vi "Off Mode Standby Mode Power Measure SM.vi"(0 "Aplus IP Address":string="192.168.1.101", 5 "Remote Port":i32=502, 11 "Error In":errorcluster) -> (2 "Complete?":bool, 4 "Off Mode Watts":dbl, 6 "2015 Output":bool, 8 "Standby Watts":dbl, 10 "Low Power Switch":bool=TRUE, 15 "Error Out":errorcluster)   [LabVIEW 2012]
uses:
  <vilib>/Analysis/NI_AALBase.lvlib
panel:
  in  "Main Tab":enum32{"Collecting", "Analyzed"}(tab)
  in  "stop":bool
  out "Power Chart":dbl(graph)
  out "Power (Watts)":dbl format="%#.2g"
  in  "Skip Standby":bool
  in  "2015 DOE":bool
  out "Off Mode Watts":T1(graph)
  out "5% of Max.":dbl
  out "Max Value.":dbl
  out "Standard Deviation.":dbl
  out "Standby Mode Watts":T1(graph)
  out "Standard Deviation":dbl
  out "Max Value":dbl
  out "5% of Max":dbl
  in  "Complete Test":bool
  in  "Restart":bool
  out "Stable?":bool
  out "Time Sum 4":dbl
  out "Time Sum 3":dbl
  out "Time Sum 2":dbl
  out "Time Sum 1":dbl
  in  "Tab Control":enum32{"Input Parameters", "Debug", "Raw Data"}(tab)
  in  "Processed Data":bool
  in  "Tab Control 2":T2(tab)
  in  "10 Min Power":dbl=600.0
  in  "35 Min":dbl=2100.0
  in  "5 Min Timer":dbl=300.0
  in  "2015?":bool
  out "Current State":string
  in  "High State Timer":dbl=10.0
  out "High Power":dbl
  in  "Low State Timer (5 min)":dbl=300.0
  out "Power Threshold":dbl
  in  "Testing":bool
  in  "Test Power":dbl
  in  "Debug?":bool=TRUE
  out "Debug State":string[](array[string])
  out "DOE Data":dbl[][](array[numeric])
  out "35 Min Data":dbl[][](array[numeric])
  out "Power Threshold Array":dbl[][](array[numeric])
  out "Timer":dbl format="%<%H:%M:%S>t"
  out "String":string
  # "Measure off mode and standby mode for DOE 2015. Reference ETP 112D026 - 2015 DOE Dryer Energy"
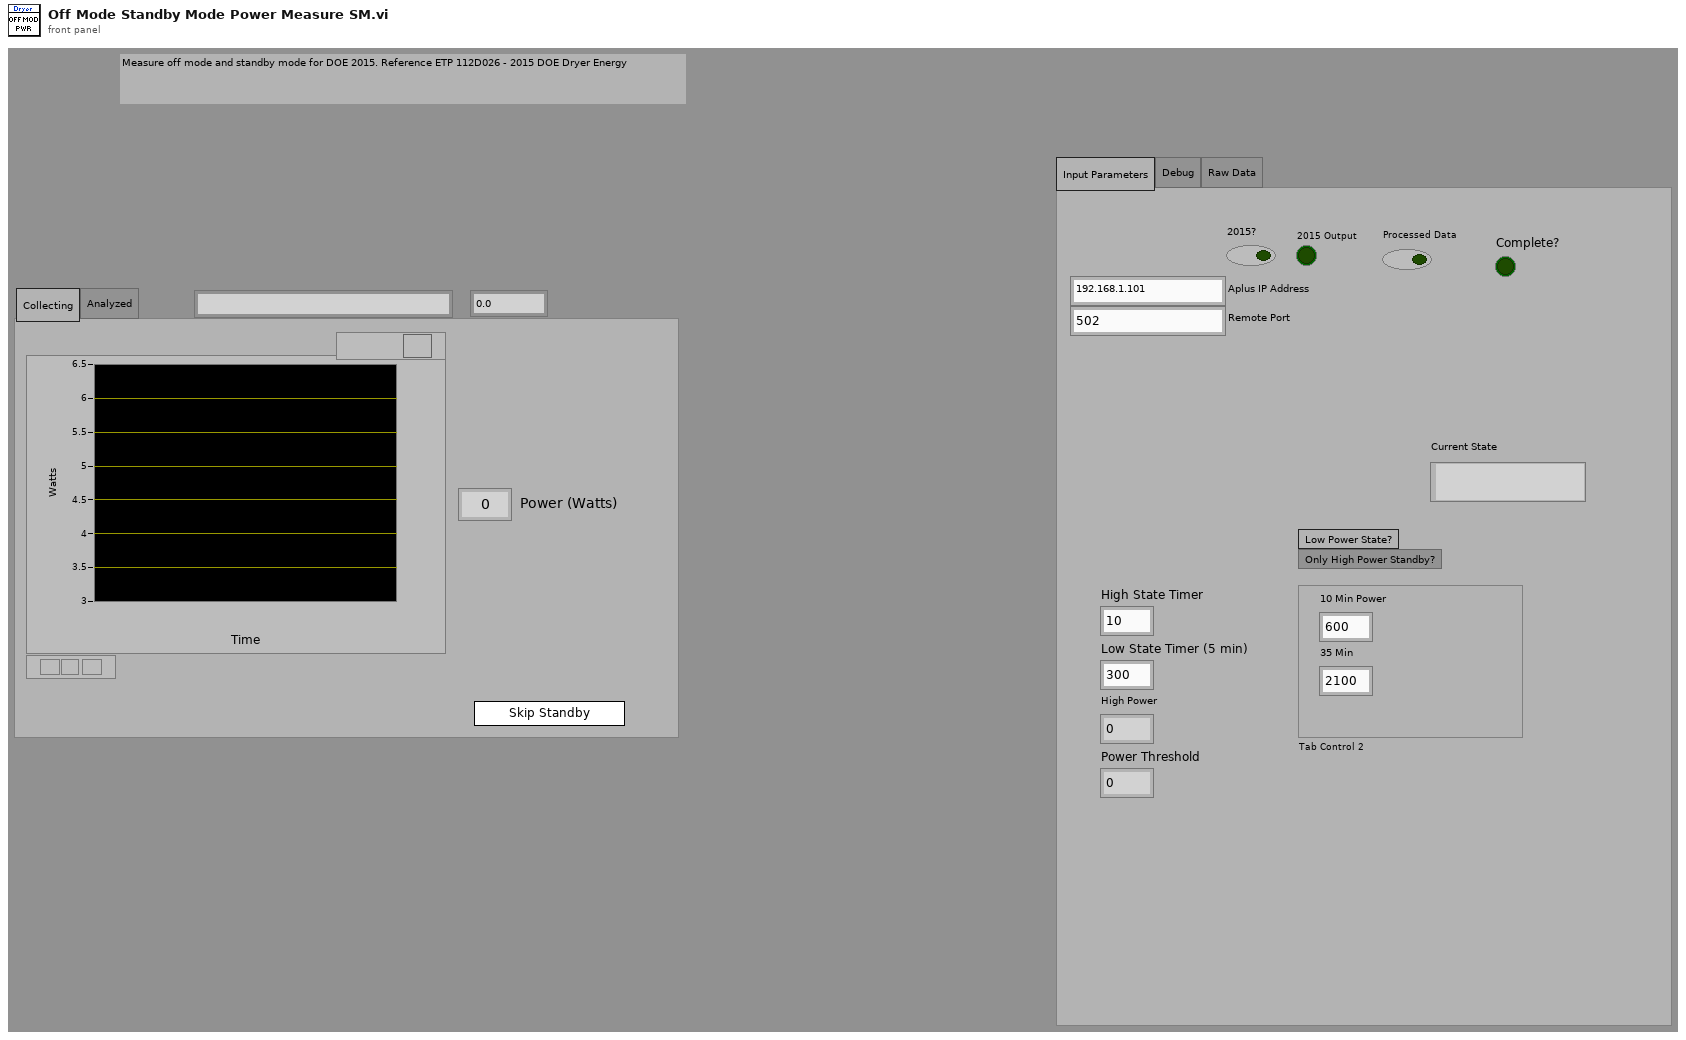
[diagram p1: front panel]
types:
  T1 = cluster{"X Values":dbl[], "Histogram: h(x)":i32[]}
  T2 = enum32{"Low Power State?", "Only High Power Standby?"}
  T3 = enum32{"invalid app kind", "Development System", "Run Time System", "Student Edition", "Embedded LabVIEW", "Evaluation", "Custom"}
  T4 = enum32{"Invalid", "Standard", "Closed", "Hidden", "Minimized", "Maximized"}
  T5 = cluster{"Core":cluster{"Current VI Reference":refnum<vi>, "Close Panel on Exit?":bool}, "Agilent Channel List":string, "T0":dbl, "Tstart":dbl, "Temps":dbl[], "2015?":bool, "Labels":string[], "35 Min Data Array":dbl[], "10 Min Data Array":dbl[], "Low Power State?":bool, "Output Data":cluster{"Standard Deviation":dbl, "Off Mode Watts":dbl, "Max Value":dbl, "5% of Max":dbl, "Standby Watts":dbl, "Standard Deviation.":dbl, "Max Value.":dbl, "5% of Max.":dbl}, "Power Threshold":dbl[], "Processed Data":bool, "Main Tab":enum32{"Collecting", "Analyzed"}, "Remote Port":i32, "Aplus IP Address":string}
  T6 = cluster{"Standard Deviation":dbl, "Off Mode Watts":dbl, "Max Value":dbl, "5% of Max":dbl, "Standby Watts":dbl, "Standard Deviation.":dbl, "Max Value.":dbl, "5% of Max.":dbl}
  T7 = cluster{"Current VI Reference":refnum<vi>, "Close Panel on Exit?":bool}
  T8 = cluster{"Voltage":sgl, "Current":sgl, "Frequency":sgl, "Power":sgl, "Power Factor":sgl, "WattHours":sgl}
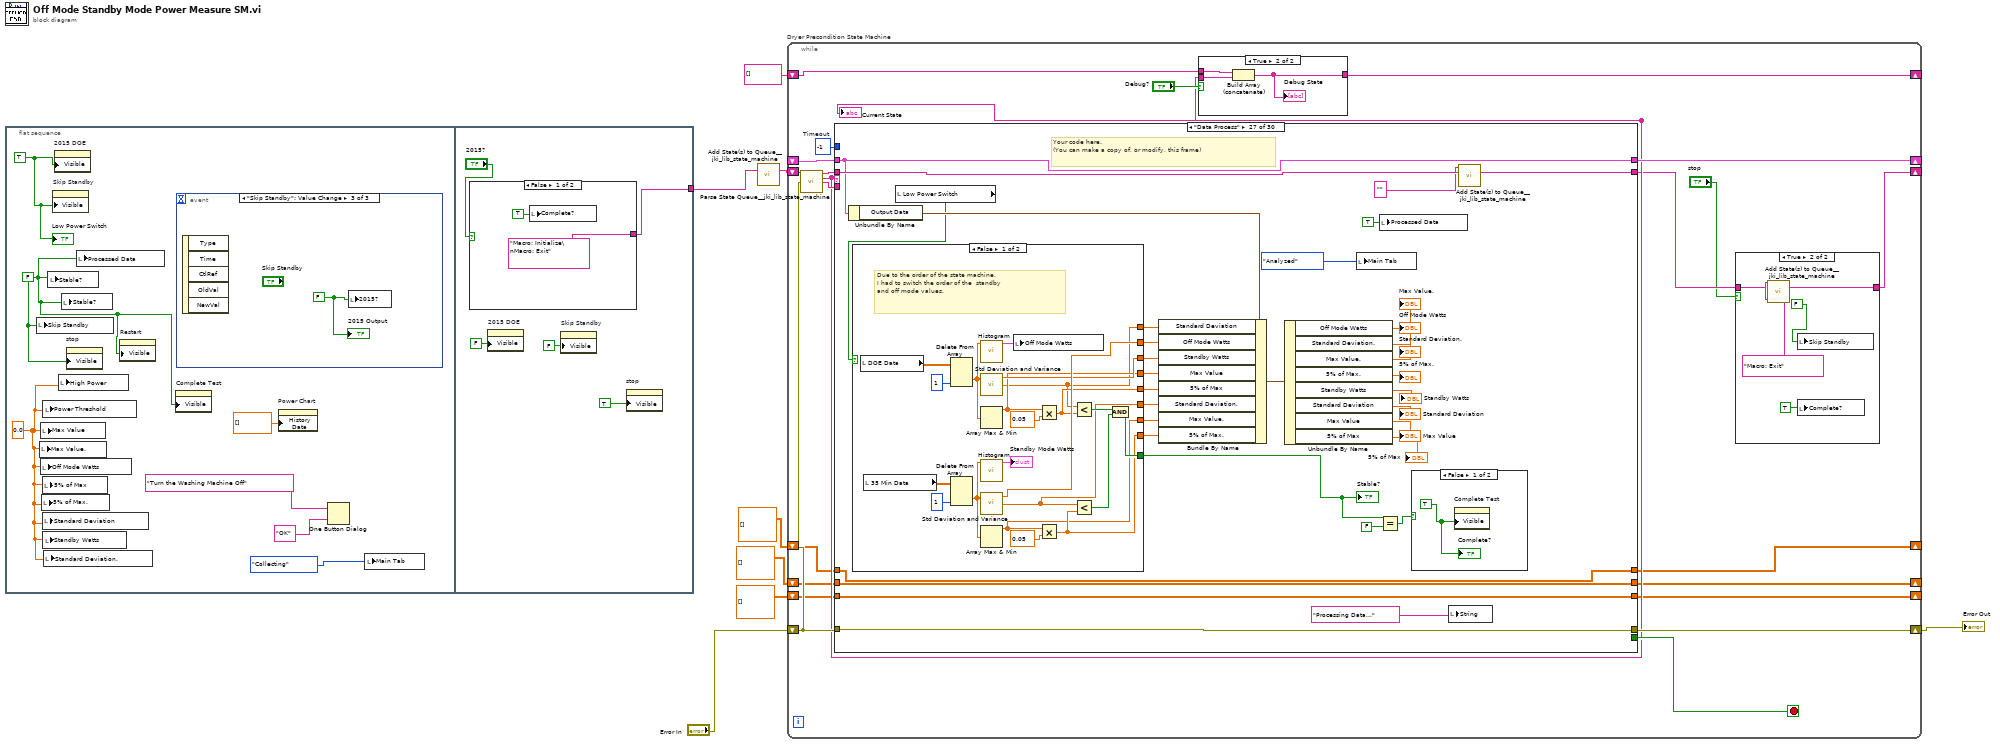
[diagram p0: block diagram]
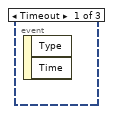
[diagram p2: hidden frame]
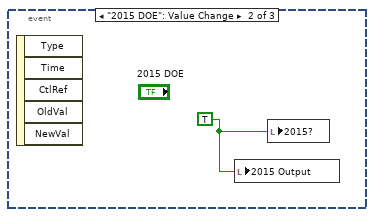
[diagram p3: hidden frame]
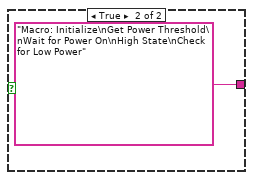
[diagram p4: hidden frame]
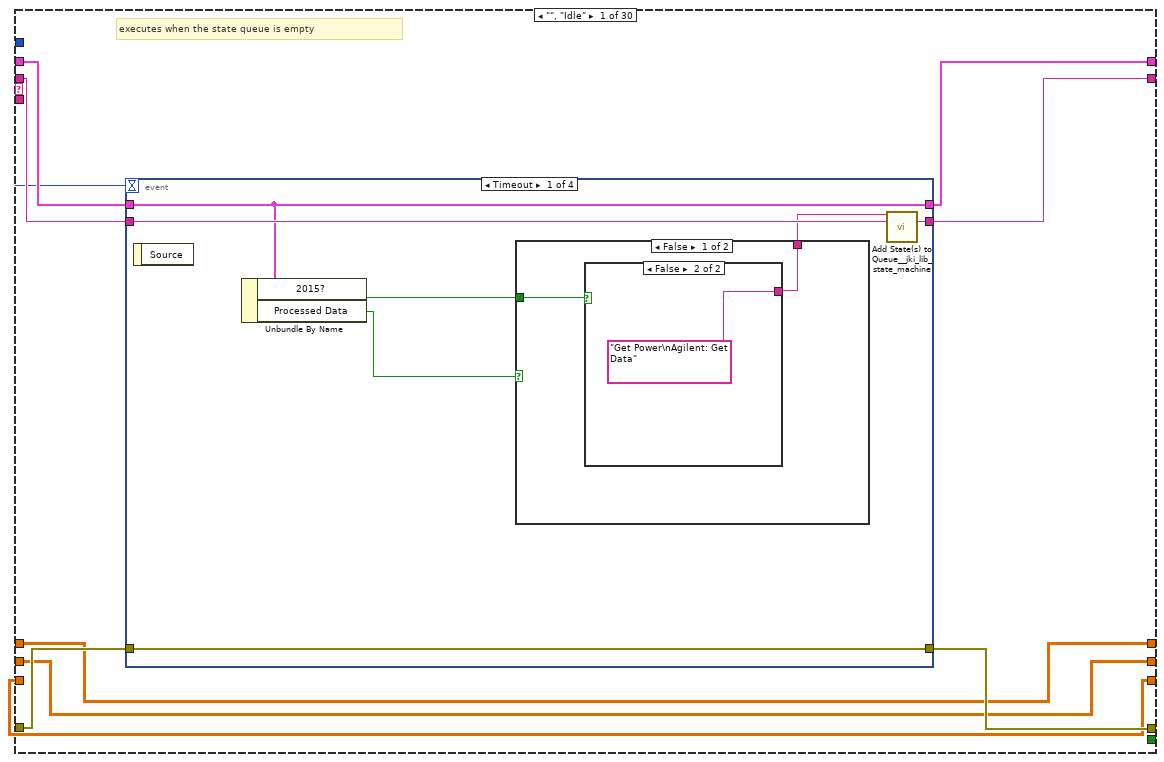
[diagram p7: hidden frame]
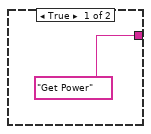
[diagram p8: hidden frame]
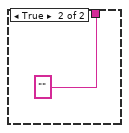
[diagram p9: hidden frame]
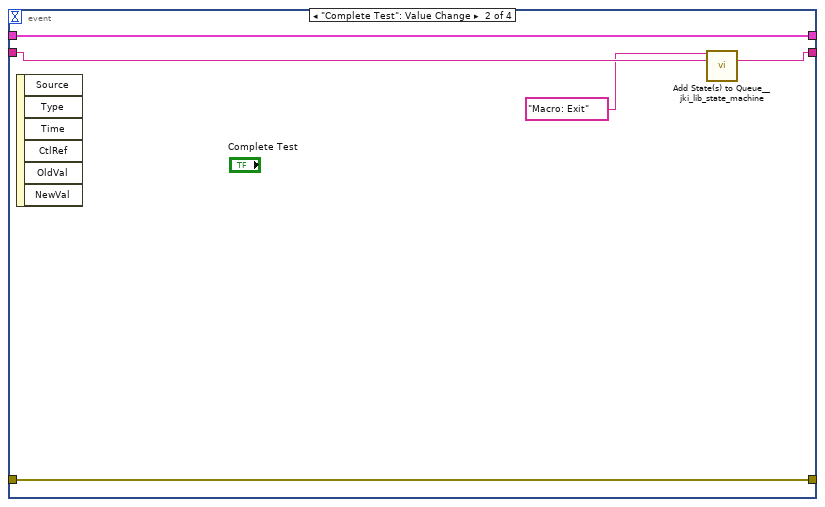
[diagram p10: hidden frame]
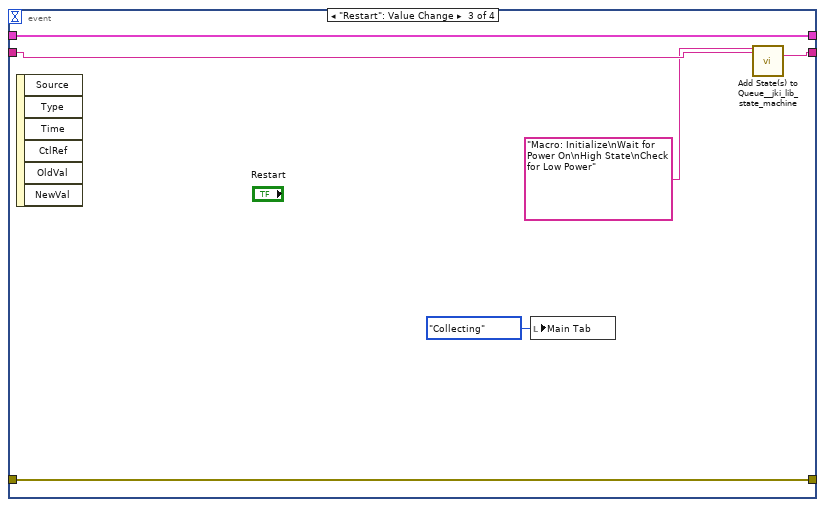
[diagram p11: hidden frame]
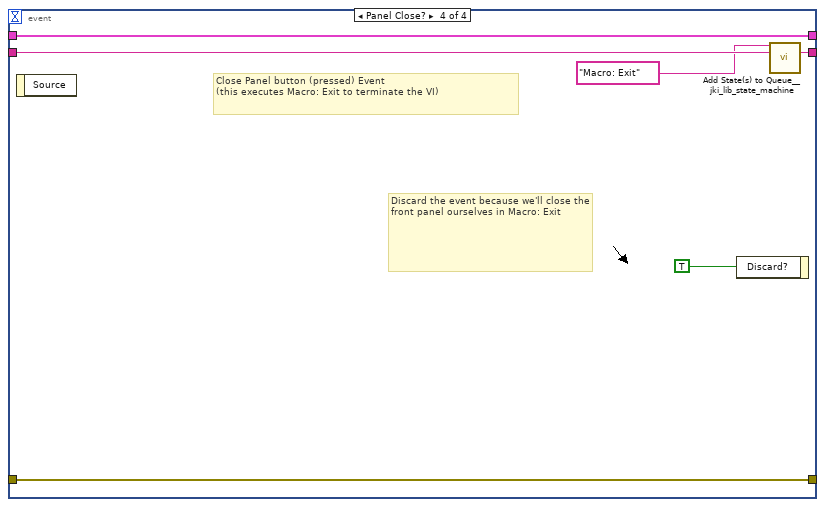
[diagram p12: hidden frame]
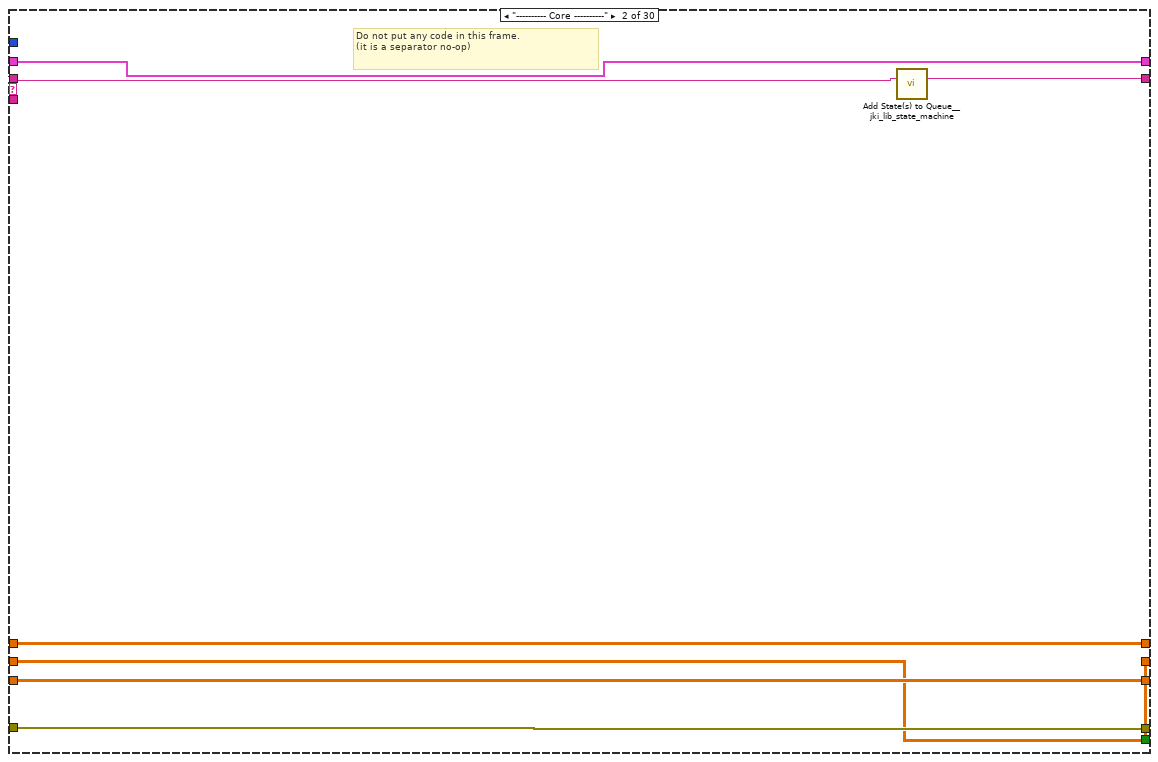
[diagram p13: hidden frame]
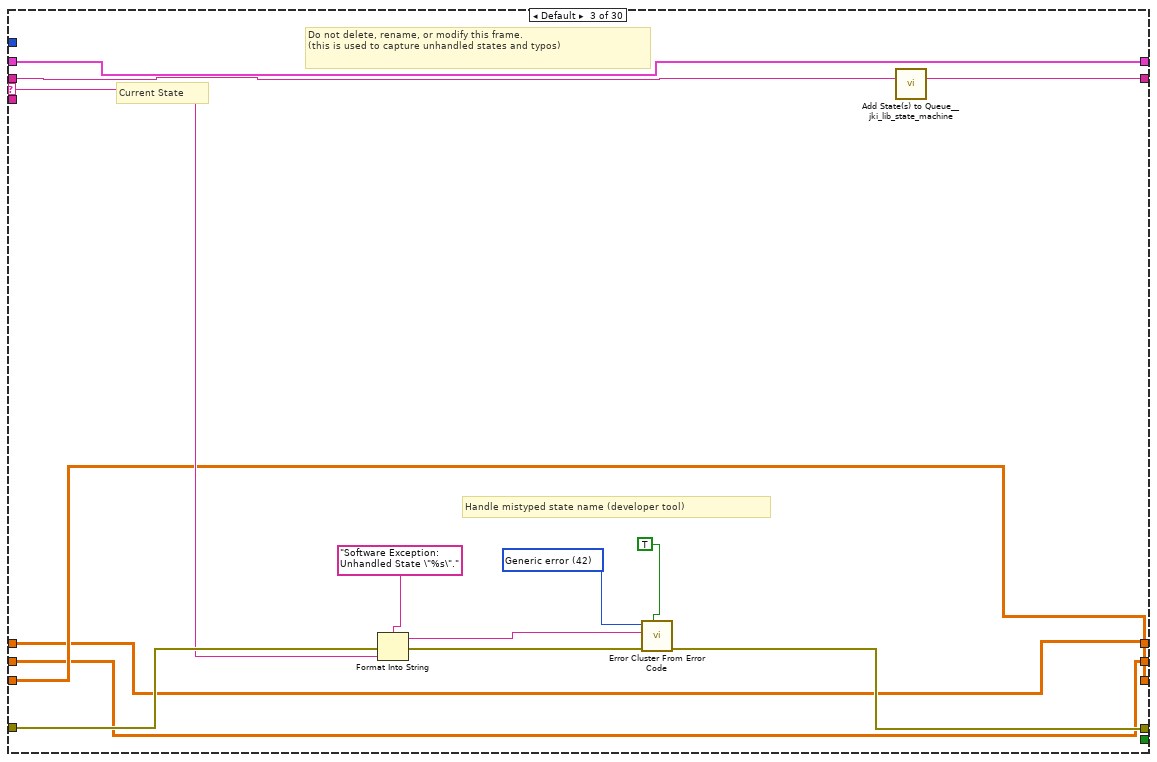
[diagram p14: hidden frame]
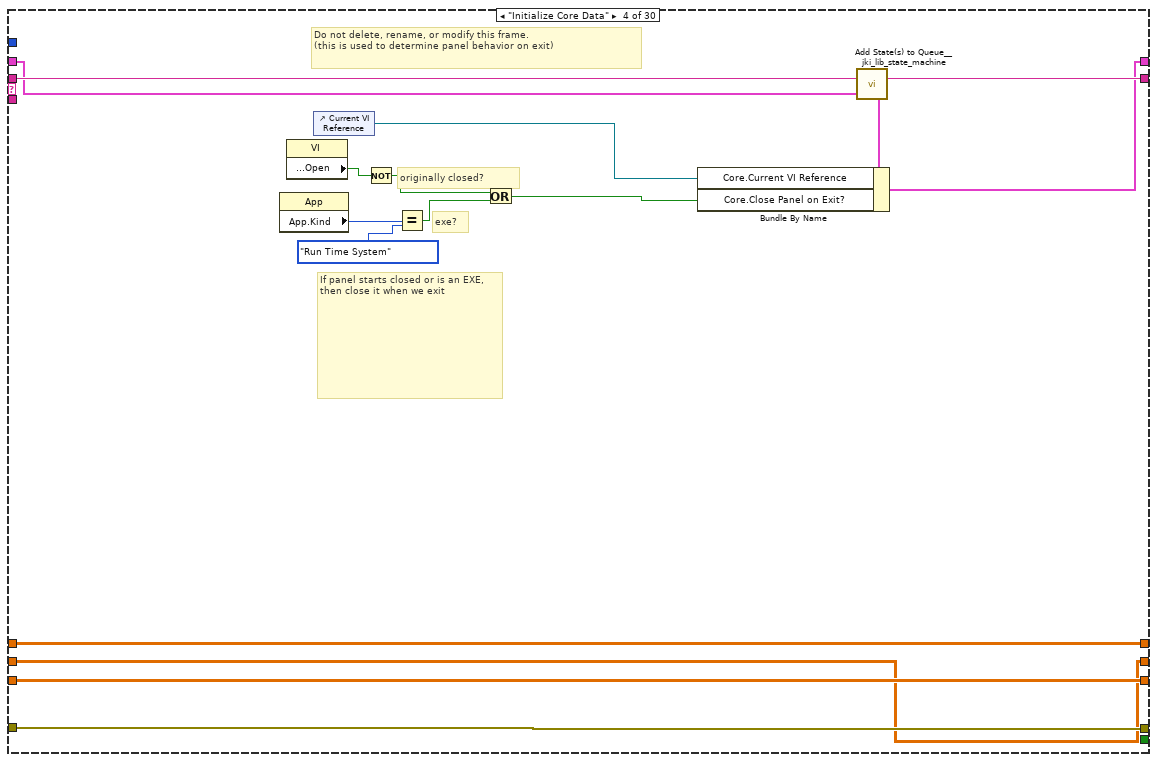
[diagram p15: hidden frame]
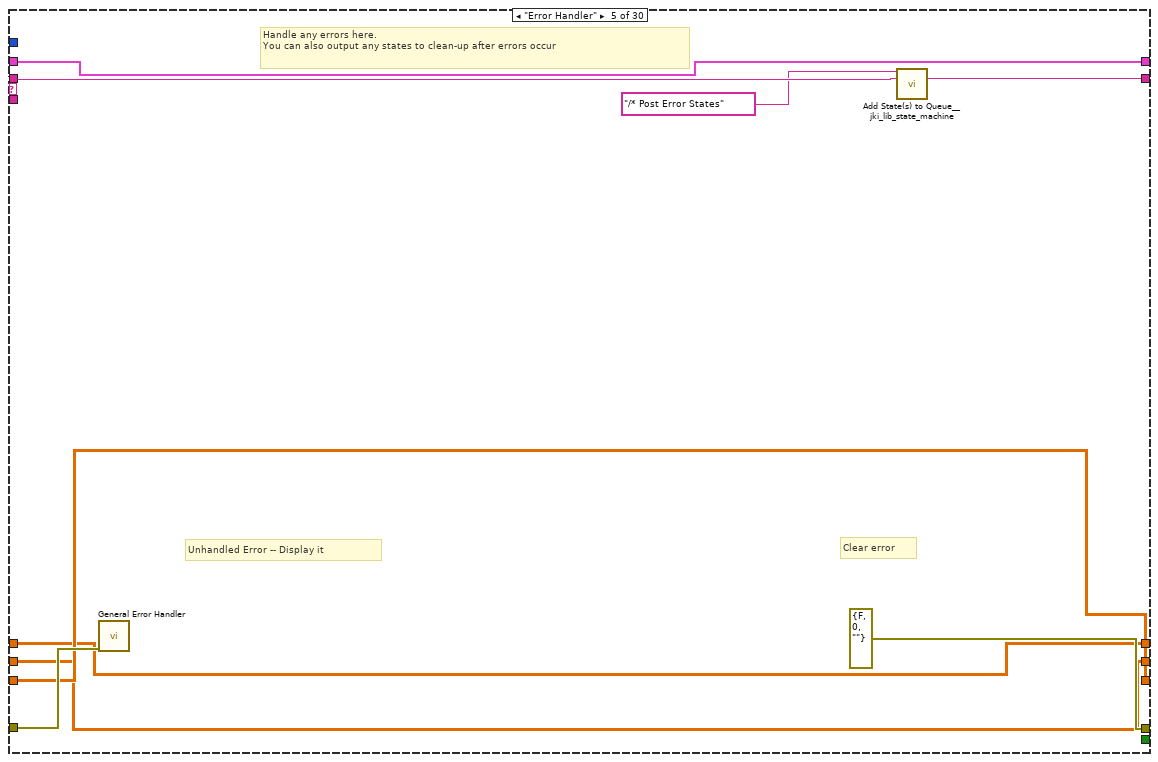
[diagram p16: hidden frame]
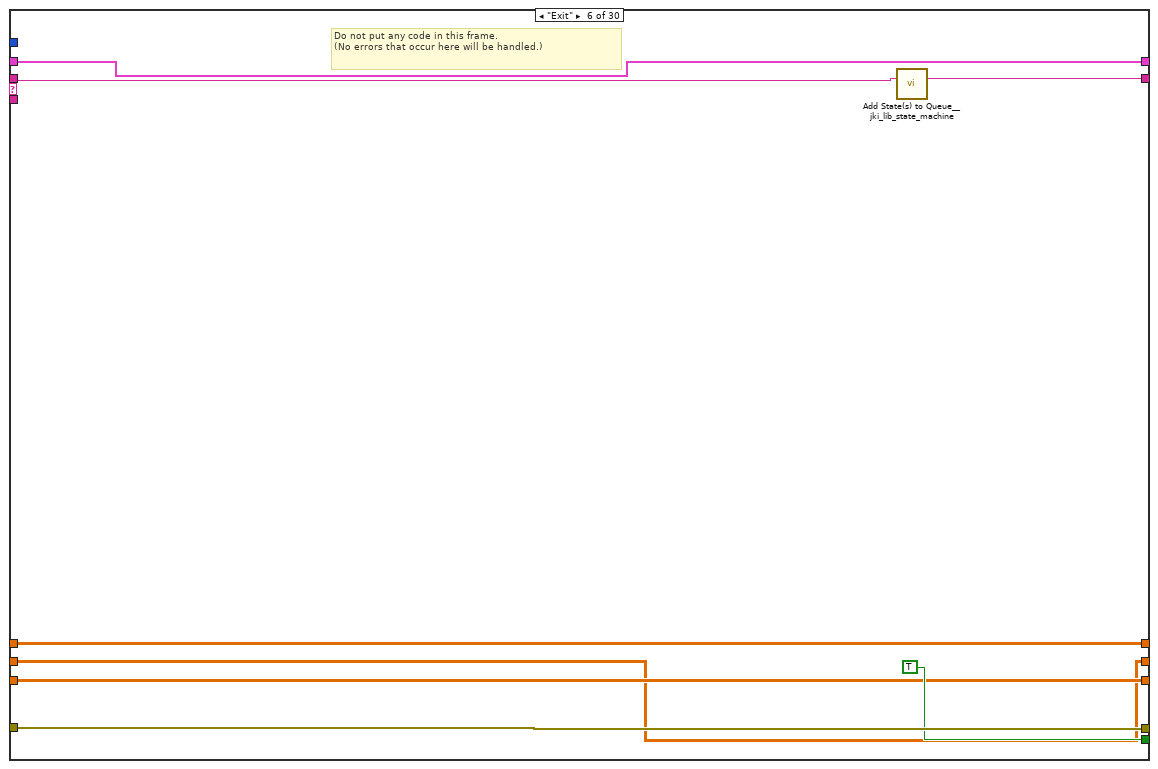
[diagram p17: hidden frame]
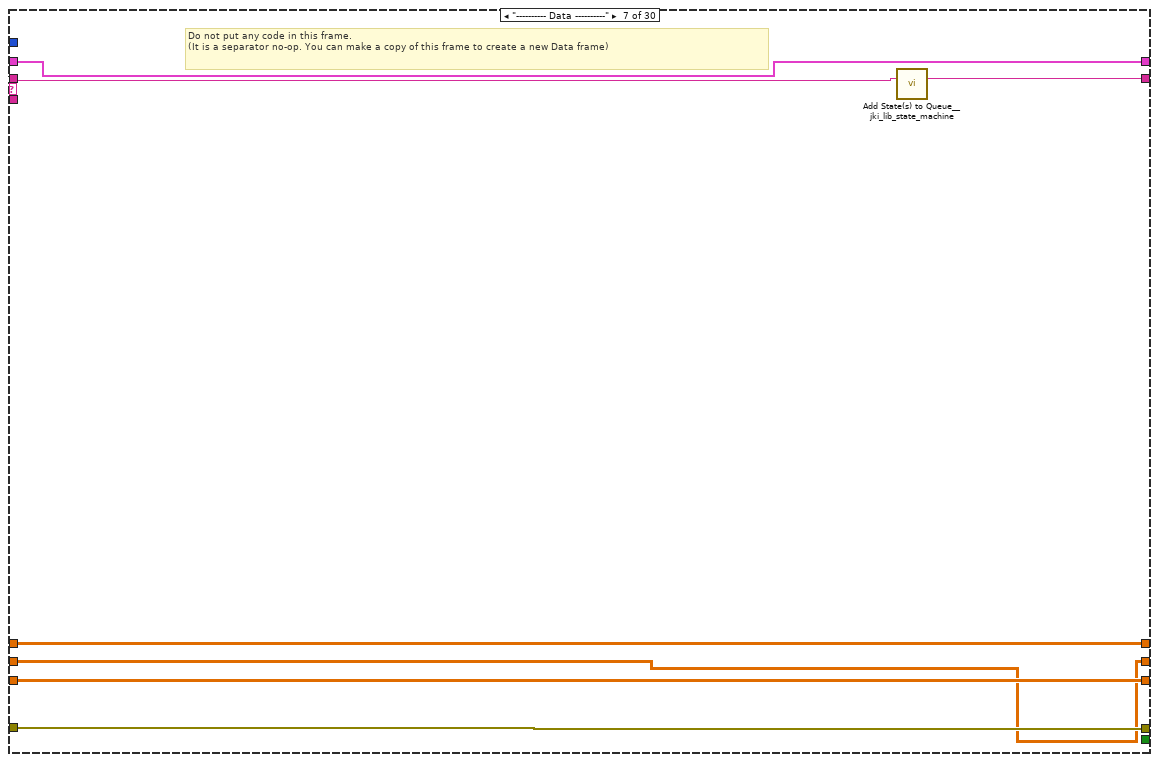
[diagram p18: hidden frame]
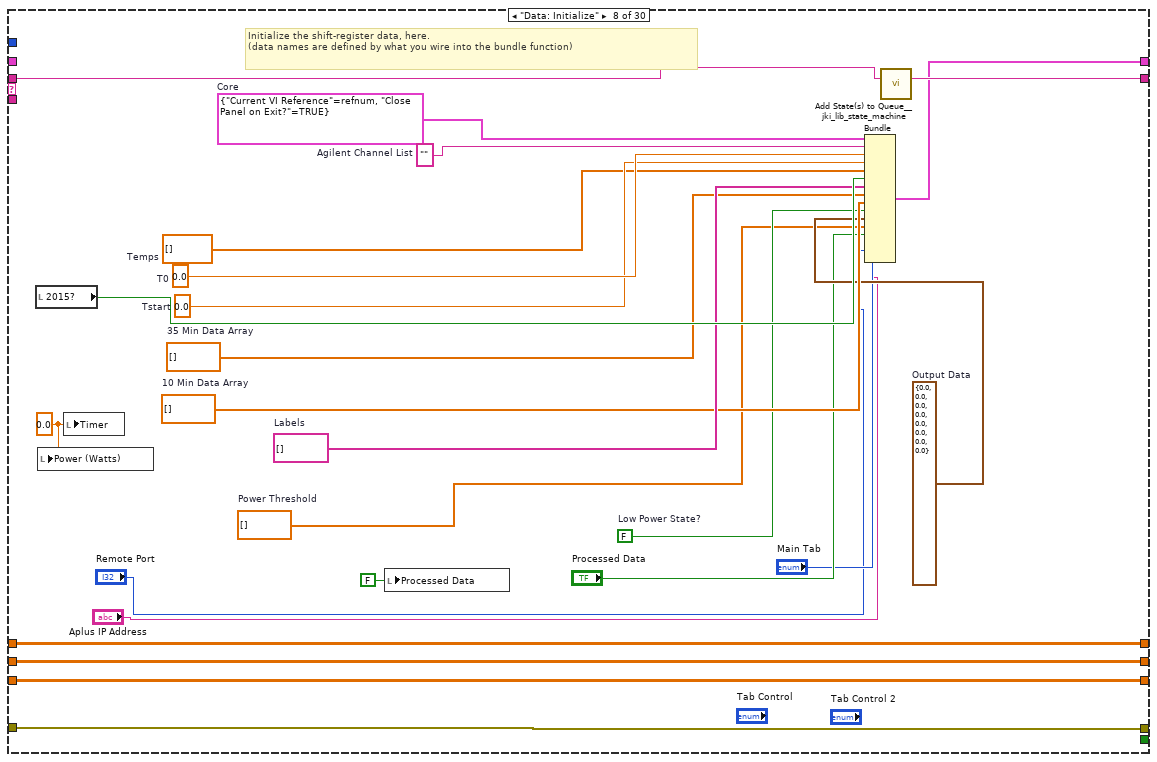
[diagram p19: hidden frame]
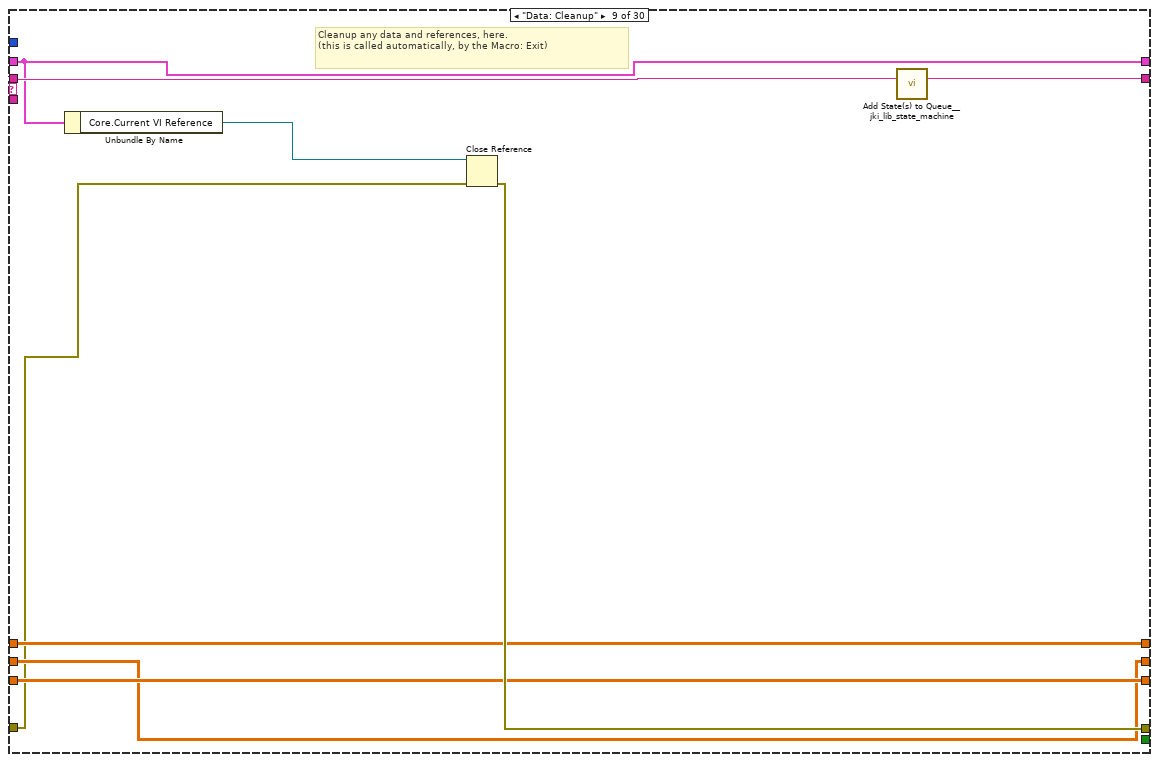
[diagram p20: hidden frame]
diagram:
  n1 = flat-sequence {
    tunnel: [w22] -> w7
    frame #0 {
      w12 = 0.0 ("Max Value")
      w10 = FALSE ("Off Mode Stable?")
      w11 = TRUE ("Visible")
      n2 = local write "Skip Standby"(w10) -> ()
      n3 = local write "Max Value."(w12) -> ()
      n4 = local write "Max Value"(w12) -> ()
      n5 = local write "Off Mode Watts"(w12) -> ()
      n6 = local write "5% of Max."(w12) -> ()
      n7 = local write "5% of Max"(w12) -> ()
      n8 = local write "Standard Deviation"(w12) -> ()
      n9 = local write "Power Threshold"(w12) -> ()
      n10 = local write "Standby Watts"(w12) -> ()
      n11 = local write "Standard Deviation."(w12) -> ()
      n12 = local write "Stable?"(w10) -> ()
      n13 = property on="Skip Standby" class="Bool (strict)"("Visible"=w11) -> ()  [unwired: 2 in, 2 out]
      n14 = property on="2015 DOE" class="Bool (strict)"("Visible"=w11) -> ()  [unwired: 2 in, 2 out]
      n15 = local write "High Power"(w12) -> ()
      n16 = local write "Stable?"(w10) -> ()
      n17 = property on="stop" class="Bool (strict)"("Visible"=w10) -> ()  [unwired: 2 in, 2 out]
      n18 = local write "Processed Data"(w10) -> ()
      n19 = property on="Restart" class="Bool (strict)"("Visible"=w10) -> ()  [unwired: 2 in, 2 out]
      n20 = property on="Complete Test" class="Bool (strict)"("Visible"=w10) -> ()  [unwired: 2 in, 2 out]
      n21 = event shown="[2] \"Skip Standby\": Value Change" {
        selector: _ -> [_ _ _]
        dyn-events: _ -> [_ _ _]
        timeout: _ -> [_ _ _]
        event Timeout {
          n22 = event-data() -> ()  [unwired: 1 in, 2 out]
        }
        event "2015 DOE": Value Change {
          w16 = TRUE ("CDAQ?")
          n23 = event-data() -> ()  [unwired: 1 in, 5 out]
          n24 = local write "2015 Output"(w16) -> ()
          n25 = local write "2015?"(w16) -> ()
        }
        event "Skip Standby": Value Change {
          w17 = FALSE ("2015?")
          n26 = event-data() -> ()  [unwired: 1 in, 5 out]
          n27 = local write "2015?"(w17) -> ()
          "2015 Output" <- w17
        }
      }
      n28 = property on="Power Chart" class="WFChart (strict)"("History Data"=dbl[] []) -> ()  [unwired: 2 in, 2 out]
      n29 = One Button Dialog(message="Turn the Washing Machine Off", button name ("OK")="OK") -> ()  [unwired: 1 out]
      n30 = local write "Main Tab"(enum32{"Collecting", "Analyzed"}."Collecting" ("Tab Control 3")) -> ()
      "Low Power Switch" <- w11
    }
    frame #1 {
      n31 = case shown="False" "2015?" {
        tunnel: ["Macro: Initialize\nMacro: Exit" "Macro: Initialize\nGet Power Threshold\nWait for Power On\nHigh State\nCheck for Low Power"] -> w22
        frame False {
          n32 = local write "Complete?"(TRUE ("Complete?")) -> ()
        }
        frame True {
        }
      }
      n33 = property on="2015 DOE" class="Bool (strict)"("Visible"=FALSE) -> ()  [unwired: 2 in, 2 out]
      n34 = property on="Skip Standby" class="Bool (strict)"("Visible"=FALSE) -> ()  [unwired: 2 in, 2 out]
      n35 = property on="stop" class="Bool (strict)"("Visible"=TRUE) -> ()  [unwired: 2 in, 2 out]
    }
  }
  n36 = call <vilib>:"Add State(s) to Queue__jki_lib_state_machine.vi"("State(s) in (\"\")"=w7) -> ("States Out"=w8:string)  [unwired: 14 in]
  n37 = while "Dryer Precondition State Machine" {
    shift-right: [w42] -> _
    shift-left: _ -> [w41]
    shift-right: [w44] -> w5
    shift-left: "Error In" -> [w39]
    shift-right: [w29] -> _
    shift-left: w8 -> [w45]
    shift-right: [w36] -> _
    shift-left: string[] [] -> [w35]
    shift-right: [w33] -> _
    shift-left: dbl[][] [] -> [w34]
    shift-right: [w31] -> _
    shift-left: dbl[][] [] -> [w32]
    shift-right: [w27] -> _
    shift-left: dbl[][] [] -> [w28]
    stop <- w43 stop-if-true
    w40 = -1  # Timeout
    n38 = call <vilib>:"Parse State Queue__jki_lib_state_machine.vi"("State Queue"=w45, "Error In (no error)"=w39) -> ("Remaining States"=w47:string, "Current State"=w37:string, "Arguments"=w46:string)  [unwired: 11 in]
    "Current State" <- w37
    n39 = case shown="\"Data Process\"" w37 {
      selector: w37 -> [_ _ w107 _ _ _ _ _ _ _ _ _ _ _ _ _ _ _ _ _ _ _ _ _ _ _ _ _ _ _]
      tunnel: w47 -> [w67 w103 w111 w132 w141 w149 w156 w181 w190 w197 w204 w213 w227 w256 w264 w277 w284 w301 w343 w377 w414 w461 w501 w538 w575 w612 w662 w706 w726 w746]
      tunnel: w46 -> [_ _ _ _ _ _ _ _ _ _ _ w208 w221 _ _ _ _ _ _ _ _ _ _ _ _ _ _ _ _ _]
      tunnel: w41 -> [w65 w100 w109 w123 w138 w147 w153 _ w186 w194 w202 w211 w223 w253 w261 w274 w281 w298 w340 w374 w411 w458 w498 w535 w572 w609 w631 w701 w724 w741]
      tunnel: [w64 w101 w113 w129 errorcluster {"status"=FALSE, "code"=0, "source"=""} ("error out") w146 w154 w179 w187 w195 w201 w209 w224 w254 w262 w275 w282 w299 w329 w375 w412 w459 w499 w536 w573 w610 w660 w702 w717 w742] -> w44
      tunnel: w39 -> [w63 w101 w112 w129 w137 w146 w154 w179 w182 w195 w201 w210 w225 w254 w262 w275 w282 w299 w329 w375 w412 w459 w499 w536 w573 w610 w660 w700 w718 w742]
      tunnel: [w66 w102 w110 w131 w140 w148 w155 w180 w189 w196 w203 w212 w226 w255 w263 w276 w283 w300 w342 w376 w413 w460 w500 w537 w574 w611 w661 w705 w725 w745] -> w30
      tunnel: [_ _ _ _ _ TRUE _ _ _ _ _ _ _ _ _ _ _ _ _ _ _ _ _ _ _ _ _ _ _ _] -> w43
      tunnel: [w62 w100 w109 w130 w138 w147 w153 w176 w186 w194 w202 w211 w223 w253 w261 w274 w281 w297 w339 w373 w410 w457 w497 w534 w571 w608 w631 w704 w723 w740] -> w42
      tunnel: w40 -> [w61 _ _ _ _ _ _ _ _ _ _ _ _ _ _ _ _ _ _ _ _ _ _ _ _ _ _ _ _ _]
      tunnel: w34 -> [w60 w99 w106 w120 w135 w144 w152 w170 w185 w193 w200 w207 w220 w252 w259 w267 w280 w287 w333 w363 w397 w447 w488 w526 w563 w594 w658 w699 w716 w737]
      tunnel: [w60 w99 w106 w120 w135 w144 w152 w170 w185 w193 w200 w207 w220 w252 w259 w267 w280 w287 w333 w363 w397 w447 w488 w521 w561 w594 w658 w699 w716 w737] -> w33
      tunnel: w32 -> [w59 w98 w105 w119 w134 w143 w151 w167 w184 w192 w199 w206 w219 w251 w258 w266 w279 w289 w332 w365 w402 w443 w486 w524 w560 w599 w657 w698 w715 w736]
      tunnel: [w59 w98 w105 w119 w134 w143 w151 w167 w184 w192 w199 w206 w219 w251 w258 w266 w279 w289 w332 w365 w402 w446 w486 w524 w560 w598 w657 w698 w715 w736] -> w31
      tunnel: w28 -> [w58 w97 w104 w118 w133 w142 w150 w162 w183 w191 w198 w205 w218 w250 w257 w265 w278 w286 w331 w362 w396 w442 w484 w519 w556 w593 w636 w697 w712 w735]
      tunnel: [w58 w97 w104 w118 w133 w142 w150 w162 w183 w191 w198 w205 w218 w250 w257 w265 w278 w285 w331 w362 w396 w442 w484 w519 w556 w593 w636 w697 w712 w735] -> w27
      frame "", "Idle" {
        # "executes when the state queue is empty"
        n40 = event shown="[0] Timeout" {
          selector: _ -> [_ _ _ _]
          dyn-events: _ -> [_ _ _ _]
          timeout: w61 -> [_ _ _ _]
          tunnel: w67 -> [w74 w83 w88 w96]
          tunnel: [w73 w81 w89 w95] -> w66
          tunnel: w65 -> [w70 w84 w90 w93]
          tunnel: [w72 w80 w86 w94] -> w64
          tunnel: w63 -> [w72 w80 w86 w94]
          tunnel: [w70 w84 w90 w93] -> w62
          event Timeout {
            n41 = event-data() -> ()  [unwired: 1 in, 1 out]
            n42 = Unbundle By Name(w70) -> ("2015?"=w69:bool, "Processed Data"=w68:bool)
            n43 = case shown="False" w68 {
              tunnel: [w76 "" ("State(s) in Front (\"\")")] -> w71
              tunnel: w69 -> [w75 _]
              frame False {
                n44 = case shown="False" w75 {
                  tunnel: ["Get Power" ("State(s) in Front (\"\")") "Get Power\nAgilent: Get Data" ("State(s) in Front (\"\")")] -> w76
                  frame True {
                  }
                  frame False {
                  }
                }
              }
              frame True {
              }
            }
            n45 = call <vilib>:"Add State(s) to Queue__jki_lib_state_machine.vi"("State(s) in Front (\"\")"=w71, "State(s) in (\"\")"=w74) -> ("States Out"=w73:string)  [unwired: 13 in]
          }
          event "Complete Test": Value Change {
            n46 = event-data() -> ()  [unwired: 1 in, 6 out]
            n47 = call <vilib>:"Add State(s) to Queue__jki_lib_state_machine.vi"("State(s) in Front (\"\")"="Macro: Exit", "State(s) in (\"\")"=w83) -> ("States Out"=w81:string)  [unwired: 13 in]
          }
          event "Restart": Value Change {
            n48 = event-data() -> ()  [unwired: 1 in, 6 out]
            n49 = local write "Main Tab"(enum32{"Collecting", "Analyzed"}."Collecting" ("Main Tab")) -> ()
            n50 = call <vilib>:"Add State(s) to Queue__jki_lib_state_machine.vi"("State(s) in Front (\"\")"="Macro: Initialize\nWait for Power On\nHigh State\nCheck for Low Power", "State(s) in (\"\")"=w88) -> ("States Out"=w89:string)  [unwired: 13 in]
          }
          event Panel Close? {
            # "Discard the event because we'll close the front panel ourselves in Macro: Exit"
            # "Close Panel button (pressed) Event\n(this executes Macro: Exit to terminate the VI)"
            n51 = event-data() -> ()  [unwired: 1 in, 1 out]
            n52 = event-data("Discard?"=TRUE) -> ()  [unwired: 1 in, 1 out]
            n53 = call <vilib>:"Add State(s) to Queue__jki_lib_state_machine.vi"("State(s) in Front (\"\")"="Macro: Exit", "State(s) in (\"\")"=w96) -> ("States Out"=w95:string)  [unwired: 13 in]
          }
        }
      }
      frame "---------- Core ----------" {
        # "Do not put any code in this frame.\n(it is a separator no-op)"
        n54 = call <vilib>:"Add State(s) to Queue__jki_lib_state_machine.vi"("State(s) in (\"\")"=w103) -> ("States Out"=w102:string)  [unwired: 14 in]
      }
      frame Default {
        w116 = 42 items=["No error", "Argument error", "Memory is full", "Out of zone", "End of file", "File already open", "Generic file I/O error", "File not found", "File permission error", "Disk is full", "Duplicate path", "Too many files open", "System feature not enabled", "Resource file not found", "Cannot add resource", "Resource not found", "Image not found", "Image memory error", "Pen does not exist", "Config type invalid", "Config token not found", "Config parse error", "Config memory error", "Bad external code format", "Bad external code offset", "External code not present", "Null window", "Destroy window error", "Null menu", "Print aborted", "Bad print record", "Print driver error", "Windows error during printing", "Memory error during printing", "Print dialog error", "Generic print error", "Invalid device refnum", "Device not found", "Device parameter error", "Device unit error", "Cannot open device", "Device call aborted", "Generic error", "Cancelled by user", "Object ID too low", "Object ID too high", "Object not in heap", "Unknown heap", "Unknown object (invalid DefProc)", "Unknown object (DefProc not in table)", "Message out of range", "Invalid (null) method", "Unknown message", "Manager call not supported", "Bad address", "Network operation in progress", "Network operation timed out", "Connection is busy", "Network attribute not supported", "Network error", "Address in use", "System out of memory", "Connection aborted", "Connection refused", "Not connected", "Already connected", "Connection closed", "Initialization error (interapplication manager)", "Bad occurrence", "Wait on unbound occurrence handler", "Occurrence queue overflow", "Datalog type conflict", "Unused", "Unrecognized type (interapplication manager)", "Memory corrupt", "Failed to make temporary DLL", "Old CIN version", "Drag socket not found", "Failed to load drop-object", "Failed to register OLE object", "Failed to release OLE object", "Format specifier type mismatch", "Unknown format specifier", "Too few format specifiers", "Too many format specifiers", "Scan failed", "Newer CIN version", "Error converting to variant", "Runtime menu error", "Password tampered", "Variant attribute not found", "Incompatible variant data type", "Event data is not available", "Event Store is not present", "Occurrence is not found", "Event Queue is not created", "Event info is not available", "Refnum passed is NULL", "Error retrieving Class GUID", "Error retrieving CoClass GUID", "Error retrieving TypeLib GUID.", "Bad built application magic bytes.", "Specific driver is different from the specific driver associated with the Logical Name.", "There is no session opened to the class driver.", "Max Error", "MAX - Error with config objects", "MAX - Error loading configuration", "MAX - Group not supported"]
        # "Current State"
        # "Do not delete, rename, or modify this frame.\n(this is used to capture unhandled states and typos)"
        # "Handle mistyped state name (developer tool)"
        n55 = Format Into String(format string="Software Exception: Unhandled State \"%s\"." ("message"), error in=w112, w107) -> (resulting string=w115:string, error out=w114:errorcluster)  [unwired: 1 in]
        n56 = call <vilib>:"Error Cluster From Error Code.vi"("show call chain? (False)"=TRUE, "error in (no error)"=w114, "error message (\"\")"=w115, "error code (0)"=w116) -> ("error out"=w113:errorcluster)  [unwired: 5 in]
        n57 = call <vilib>:"Add State(s) to Queue__jki_lib_state_machine.vi"("State(s) in (\"\")"=w111) -> ("States Out"=w110:string)  [unwired: 14 in]
      }
      frame "Initialize Core Data" {
        # "Do not delete, rename, or modify this frame.\n(this is used to determine panel behavior on exit)"
        # "originally closed?"
        # "exe?"
        # "If panel starts closed or is an EXE, then close it when we exit"
        n58 = property class="App"() -> ("App.Kind"=w127:T3)  [unwired: 2 in, 2 out]
        n59 = property class="VI"() -> ("Front Panel.Open"=w128:bool)  [unwired: 2 in, 2 out]
        n60 = control-ref of="Current VI Reference"() -> (w121:refnum<vi>)
        n61 = Not(x=w128) -> (.not. x?=w125:bool)
        n62 = Equal?(x=w127, y=T3."Run Time System" ("Application:Kind")) -> (x = y?=w124:bool)
        n63 = Or(x=w125, y=w124) -> (x .or. y?=w122:bool)
        n64 = Bundle By Name(cluster=w123, "Core.Current VI Reference"=w121, "Core.Close Panel on Exit?"=w122) -> (w130:T5)
        n65 = call <vilib>:"Add State(s) to Queue__jki_lib_state_machine.vi"("State(s) in (\"\")"=w132) -> ("States Out"=w131:string)  [unwired: 14 in]
      }
      frame "Error Handler" {
        # "Unhandled Error -- Display it"
        # "Handle any errors here.\nYou can also output any states to clean-up after errors occur"
        # "Clear error"
        n66 = call <vilib>:"General Error Handler.vi"("error in (no error)"=w137) -> ()  [unwired: 10 in, 5 out]
        n67 = call <vilib>:"Add State(s) to Queue__jki_lib_state_machine.vi"("State(s) in Front (\"\")"="/* Post Error States", "State(s) in (\"\")"=w141) -> ("States Out"=w140:string)  [unwired: 13 in]
      }
      frame "Exit" {
        # "Do not put any code in this frame.\n(No errors that occur here will be handled.)"
        n68 = call <vilib>:"Add State(s) to Queue__jki_lib_state_machine.vi"("State(s) in (\"\")"=w149) -> ("States Out"=w148:string)  [unwired: 14 in]
      }
      frame "---------- Data ----------" {
        # "Do not put any code in this frame.\n(It is a separator no-op. You can make a copy of this frame to create a new Data frame)"
        n69 = call <vilib>:"Add State(s) to Queue__jki_lib_state_machine.vi"("State(s) in (\"\")"=w156) -> ("States Out"=w155:string)  [unwired: 14 in]
      }
      frame "Data: Initialize" {
        w163 = dbl[] []  # Power Threshold
        w164 = T6 {"Standard Deviation"=0.0, "Off Mode Watts"=0.0, "Max Value"=0.0, "5% of Max"=0.0, "Standby Watts"=0.0, "Standard Deviation."=0.0, "Max Value."=0.0, "5% of Max."=0.0}  # Output Data
        w165 = FALSE  # Low Power State?
        w166 = 0.0 ("Timer")
        w168 = dbl[] []  # 10 Min Data Array
        w169 = dbl[] []  # 35 Min Data Array
        w171 = string[] []  # Labels
        w173 = dbl[] []  # Temps
        w174 = 0.0  # Tstart
        w175 = 0.0  # T0
        w177 = ""  # Agilent Channel List
        w178 = T7 {"Current VI Reference"=refnum, "Close Panel on Exit?"=TRUE}  # Core
        # "Initialize the shift-register data, here.\n(data names are defined by what you wire into the bundle function)"
        n70 = local read "2015?"() -> (w172:bool)
        n71 = local write "Power (Watts)"(w166) -> ()
        n72 = local write "Timer"(w166) -> ()
        n73 = local write "Processed Data"(FALSE ("Processed Data")) -> ()
        n74 = Bundle("Core"=w178, "Agilent Channel List"=w177, "T0"=w175, "Tstart"=w174, "Temps"=w173, "2015?"=w172, "Labels"=w171, "35 Min Data Array"=w169, "10 Min Data Array"=w168, "Low Power State?"=w165, "Output Data"=w164, "Power Threshold"=w163, "Processed Data"="Processed Data", "Main Tab"="Main Tab", "Remote Port"="Remote Port", "Aplus IP Address"="Aplus IP Address") -> (w176:T5)  [unwired: 1 in]
        n75 = call <vilib>:"Add State(s) to Queue__jki_lib_state_machine.vi"("State(s) in (\"\")"=w181) -> ("States Out"=w180:string)  [unwired: 14 in]
      }
      frame "Data: Cleanup" {
        # "Cleanup any data and references, here.\n(this is called automatically, by the Macro: Exit)"
        n76 = Unbundle By Name(w186) -> ("Core.Current VI Reference"=w188:refnum<vi>)
        n77 = Close Reference(reference=w188, error in (no error)=w182) -> (error out=w187:errorcluster)
        n78 = call <vilib>:"Add State(s) to Queue__jki_lib_state_machine.vi"("State(s) in (\"\")"=w190) -> ("States Out"=w189:string)  [unwired: 14 in]
      }
      frame "---------- UI ----------" {
        # "Do not put any code in this frame.\n(It is a separator no-op. You can make a copy of this frame to create a new UI frame)"
        n79 = call <vilib>:"Add State(s) to Queue__jki_lib_state_machine.vi"("State(s) in (\"\")"=w197) -> ("States Out"=w196:string)  [unwired: 14 in]
      }
      frame "UI: Initialize" {
        # "Initialize the User Interface, here.\n(this is called automatically, by the Macro: Init)"
        n80 = call <vilib>:"Add State(s) to Queue__jki_lib_state_machine.vi"("State(s) in (\"\")"=w204) -> ("States Out"=w203:string)  [unwired: 14 in]
      }
      frame "UI: Cursor Set" {
        # "Argument"
        # "Set and Unset Cursor Busy.\n(Usage: \"UI: Cursor Set >> Busy|Idle\")"
        n81 = case shown="\"Idle\", Default" w208 {
          tunnel: w210 -> [w215 w217]
          tunnel: [w214 w216] -> w209
          frame "Idle", Default {
            n82 = call <vilib>:"Unset Busy.vi"("error in (no error)"=w215) -> ("error out"=w214:errorcluster)  [unwired: 10 in]
          }
          frame "Busy" {
            n83 = call <vilib>:"Set Busy.vi"("error in (no error)"=w217) -> ("error out"=w216:errorcluster)  [unwired: 9 in, 1 out]
          }
        }
        n84 = call <vilib>:"Add State(s) to Queue__jki_lib_state_machine.vi"("State(s) in (\"\")"=w213) -> ("States Out"=w212:string)  [unwired: 14 in]
      }
      frame "UI: Front Panel State" {
        # "Argument"
        # "Set Front Panel Open or Closed\n(Usage: \"UI: Front Panel State >> Open|Close\")"
        n85 = Unbundle By Name(w223) -> ("Core.Current VI Reference"=w222:refnum<vi>)
        n86 = case shown="\"Open\", Default" w221 {
          tunnel: w225 -> [w231 w244]
          tunnel: [w233 w245] -> w224
          tunnel: w222 -> [w232 w242]
          frame "Open", Default {
            n87 = property class="VI"(reference=w232, error in=w231) -> (reference out=w229:refnum<vi>, error out=w230:errorcluster, "Front Panel.Open"=w228:bool)
            n88 = case shown="True" w228 {
              tunnel: [w236 w239] -> w233
              tunnel: w230 -> [w235 w239]
              tunnel: w229 -> [w234 _]
              frame False {
                n89 = invoke class="VI" method="FP.Open"(reference=w234, error in=w235, "Activate"=TRUE, "State"=T4."Standard") -> (error out=w236:errorcluster)  [unwired: 1 in, 4 out]
              }
              frame True {
              }
            }
          }
          frame "Close" {
            n90 = property class="VI"(reference=w242, error in=w244) -> (reference out=w241:refnum<vi>, error out=w243:errorcluster, "Front Panel.Open"=w240:bool)
            n91 = case shown="True" w240 {
              tunnel: [w246 w249] -> w245
              tunnel: w243 -> [w246 w248]
              tunnel: w241 -> [_ w247]
              frame False {
              }
              frame True {
                n92 = invoke class="VI" method="FP.Close"(reference=w247, error in=w248) -> (error out=w249:errorcluster)  [unwired: 1 in, 2 out]
              }
            }
          }
        }
        n93 = call <vilib>:"Add State(s) to Queue__jki_lib_state_machine.vi"("State(s) in (\"\")"=w227) -> ("States Out"=w226:string)  [unwired: 14 in]
      }
      frame "---------- Macro ----------" {
        # "Do not put any code in this frame.\n(It is a separator no-op. You can make a copy of this frame to create a new Macro frame)"
        n94 = call <vilib>:"Add State(s) to Queue__jki_lib_state_machine.vi"("State(s) in (\"\")"=w256) -> ("States Out"=w255:string)  [unwired: 14 in]
      }
      frame "Macro: Initialize" {
        w260 = "Data: Initialize\nInit: Time\nInitialize Core Data\nUI: Initialize\nUI: Front Panel State >> Open"  # Data: Initialize Init: Time Initialize Core Data UI: Initialize UI: Front Panel State >> Open
        # "Initialization Macro\n(This is called once, when the VI starts)"
        n95 = call <vilib>:"Add State(s) to Queue__jki_lib_state_machine.vi"("State(s) in Front (\"\")"=w260, "State(s) in (\"\")"=w264) -> ("States Out"=w263:string)  [unwired: 13 in]
      }
      frame "Macro: Exit" {
        # "Exit Macro\n(This is called once, when the VI exits)"
        n96 = Unbundle By Name(w274) -> ("Core.Close Panel on Exit?"=w273:bool)
        n97 = Select(t="UI: Front Panel State >> Close", s=w273, f="") -> (s? t:f=w270:string)
        n98 = call <vilib>:"Add State(s) to Queue__jki_lib_state_machine.vi"("State(s) in (\"\")"=w270, "State(s) at Back (\"\")"="Data: Cleanup\nExit") -> ("States Out"=w268:string)  [unwired: 13 in]
        n99 = call <vilib>:"Add State(s) to Queue__jki_lib_state_machine.vi"("State(s) in Front (\"\")"=w268, "State(s) in (\"\")"=w277) -> ("States Out"=w276:string)  [unwired: 13 in]
      }
      frame "----------Test ----------" {
        # "Template Separator\n(You can make a copy of, or modify, this frame)"
        n100 = call <vilib>:"Add State(s) to Queue__jki_lib_state_machine.vi"("State(s) in (\"\")"=w284) -> ("States Out"=w283:string)  [unwired: 14 in]
      }
      frame "Get Power Threshold" {
        # "Your code here.\n(You can make a copy of, or modify, this frame)"
        n101 = Unbundle By Name(w298) -> ("Tstart"=w295:dbl, "2015?"=w291:bool, "35 Min Data Array"=w290:dbl[])
        n102 = Build Array (concatenate)(w286, w290) -> (w285:dbl[][])
        "Power Threshold Array" <- w285
        n103 = local read "Timer"() -> (w293:dbl)
        n104 = Greater?(x=w293, y=30.0) -> (0:w294:bool)
        n105 = case shown="False" w294 {
          tunnel: w298 -> [w309 w319]
          tunnel: [w308 w318] -> w297
          tunnel: [w307 "" ("State(s) in Front (\"\")")] -> w296
          tunnel: w295 -> [w304 _]
          tunnel: w291 -> [w303 _]
          tunnel: w285 -> [_ w327]
          frame False {
            n106 = call "E-Time.vi"() -> ("Elapsed Time (sec)"=w310:dbl)  [unwired: 9 in, 2 out]
            n107 = call "RLT Timeout Calc.vi"("Complete time"=w310, "Gather Data Period"=1000, "Start Time"=w304) -> ("coerced(x)"=w306:i32)  [unwired: 8 in]
            n108 = event shown="[0] Timeout" {
              selector: _ -> [_]
              dyn-events: _ -> [_]
              timeout: w306 -> [_]
              tunnel: [w313] -> w302
              tunnel: [w312] -> w307
              tunnel: w303 -> [w311]
              event Timeout {
                n109 = event-data() -> ()  [unwired: 1 in, 2 out]
                n110 = case shown="True" w311 {
                  tunnel: ["Post Time\nGet Power\nGet Power Threshold" ("State(s) in Front (\"\")") "Post Time\nGet Power\nAgilent: Get Data\nWait for 5 Mins" ("State(s) in Front (\"\")")] -> w312
                  frame True {
                  }
                  frame False {
                  }
                }
                n111 = call "E-Time.vi"() -> ("Elapsed Time (sec)"=w313:dbl)  [unwired: 9 in, 2 out]
              }
            }
            n112 = Bundle By Name(cluster=w309, "Tstart"=w302) -> (w308:T5)
          }
          frame True {
            # "Set the Power Threshold at 150% of the average"
            n113 = Delete From Array(array=w327, index (col)=1 ("disabled index (col)")) -> (deleted portion=w322:dbl[])  [unwired: 2 in, 1 out]
            n114 = Delete From Array(array=w322, index=0) -> (array with subset deleted=w320:dbl[])  [unwired: 1 in, 1 out]
            n115 = call <vilib>:"Std Deviation and Variance.vi"("X"=w320) -> ("mean"=w325:dbl)  [unwired: 1 in, 2 out]
            n116 = call "E-Time.vi"("Reset"=TRUE) -> ("Elapsed Time (sec)"=w317:dbl)  [unwired: 8 in, 2 out]
            n117 = Multiply(x=w325, y=1.5) -> (x*y=→"Power Threshold":dbl)
            n118 = Bundle By Name(cluster=w319, "Tstart"=w317, "T0"=w317) -> (w318:T5)
          }
        }
        n119 = local write "String"("Calculating the Power Threshold...") -> ()
        n120 = call <vilib>:"Add State(s) to Queue__jki_lib_state_machine.vi"("State(s) in Front (\"\")"=w296, "State(s) in (\"\")"=w301) -> ("States Out"=w300:string)  [unwired: 13 in]
      }
      frame "Wait for Power On" {
        # "Your code here.\n(You can make a copy of, or modify, this frame)"
        n121 = local read "Power (Watts)"() -> (w336:dbl)
        n122 = local read "Power Threshold"() -> (w330:dbl)
        n123 = Unbundle By Name(w340) -> ("2015?"=w334:bool, "Tstart"=w337:dbl)
        n124 = Greater?(x=w330, y=w336) -> (0:w335:bool)
        n125 = case shown="True" w335 {
          tunnel: w340 -> [w346 w355]
          tunnel: [w346 w354] -> w339
          tunnel: ["" ("State(s) in Front (\"\")") w352] -> w338
          tunnel: w337 -> [_ w349]
          tunnel: w334 -> [_ w347]
          frame False {
            n126 = local write "Timer"(0.0 ("Timer")) -> ()
          }
          frame True {
            n127 = call "E-Time.vi"() -> ("Elapsed Time (sec)"=w356:dbl)  [unwired: 9 in, 2 out]
            n128 = call "RLT Timeout Calc.vi"("Complete time"=w356, "Gather Data Period"=1000, "Start Time"=w349) -> ("coerced(x)"=w351:i32)  [unwired: 8 in]
            n129 = event shown="[0] Timeout" {
              selector: _ -> [_]
              dyn-events: _ -> [_]
              timeout: w351 -> [_]
              tunnel: [w358] -> w353
              tunnel: [w359] -> w352
              tunnel: [w358] -> w348
              tunnel: w347 -> [w357]
              event Timeout {
                n130 = event-data() -> ()  [unwired: 1 in, 2 out]
                n131 = case shown="True" w357 {
                  tunnel: ["Get Power\nWait for Power On" ("State(s) in Front (\"\")") "Get Power\nAgilent: Get Data\nWait for Power On" ("State(s) in Front (\"\")")] -> w359
                  frame True {
                  }
                  frame False {
                  }
                }
                n132 = call "E-Time.vi"() -> ("Elapsed Time (sec)"=w358:dbl)  [unwired: 9 in, 2 out]
              }
            }
            n133 = Bundle By Name(cluster=w355, "Tstart"=w353, "T0"=w348) -> (w354:T5)
          }
        }
        n134 = call <vilib>:"Add State(s) to Queue__jki_lib_state_machine.vi"("State(s) in Front (\"\")"=w338, "State(s) in (\"\")"=w343) -> ("States Out"=w342:string)  [unwired: 13 in]
        "String" <- "Waiting for Power ON"
      }
      frame "High State" {
        # "Your code here.\n(You can make a copy of, or modify, this frame)"
        n135 = Unbundle By Name(w374) -> ("Tstart"=w371:dbl, "2015?"=w367:bool)
        n136 = local read "Timer"() -> (w369:dbl)
        n137 = Greater?(x=w369, y="High State Timer") -> (0:w370:bool)
        n138 = case shown="True" w370 {
          tunnel: w374 -> [w386 w395]
          tunnel: [w385 w395] -> w373
          tunnel: [w383 "" ("State(s) in Front (\"\")")] -> w372
          tunnel: w371 -> [w380 _]
          tunnel: w367 -> [w379 _]
          tunnel: string[] ["Time", "Power", "Ambient Temp (F)", "RH", "RDB (F)"] ("Array") -> [w378 _]
          frame False {
            n139 = call "E-Time.vi"() -> ("Elapsed Time (sec)"=w387:dbl)  [unwired: 9 in, 2 out]
            n140 = call "RLT Timeout Calc.vi"("Complete time"=w387, "Gather Data Period"=1000, "Start Time"=w380) -> ("coerced(x)"=w382:i32)  [unwired: 8 in]
            n141 = event shown="[0] Timeout" {
              selector: _ -> [_]
              dyn-events: _ -> [_]
              timeout: w382 -> [_]
              tunnel: [w390] -> w384
              tunnel: [w389] -> w383
              tunnel: w379 -> [w388]
              event Timeout {
                n142 = event-data() -> ()  [unwired: 1 in, 2 out]
                n143 = case shown="True" w388 {
                  tunnel: ["Post Time\nGet Power\nHigh State" ("State(s) in Front (\"\")") "Post Time\nGet Power\nAgilent: Get Data\nWait for 5 Mins" ("State(s) in Front (\"\")")] -> w389
                  frame True {
                  }
                  frame False {
                  }
                }
                n144 = call "E-Time.vi"() -> ("Elapsed Time (sec)"=w390:dbl)  [unwired: 9 in, 2 out]
              }
            }
            n145 = Bundle By Name(cluster=w386, "Tstart"=w384, "Labels"=w378) -> (w385:T5)
          }
          frame True {
            # "Set the high power state"
            n146 = local read "Power (Watts)"() -> (→"High Power":dbl)
          }
        }
        n147 = local write "String"("Recording High Power State...") -> ()
        n148 = call <vilib>:"Add State(s) to Queue__jki_lib_state_machine.vi"("State(s) in Front (\"\")"=w372, "State(s) in (\"\")"=w377) -> ("States Out"=w376:string)  [unwired: 13 in]
      }
      frame "Check for Low Power" {
        # "Your code here.\n(You can make a copy of, or modify, this frame)"
        n149 = Unbundle By Name(w411) -> ("Tstart"=w408:dbl, "2015?"=w404:bool, "Low Power State?"=w398:bool)
        n150 = local read "High State Timer"() -> (w400:dbl)
        n151 = local read "Timer"() -> (w406:dbl)
        n152 = Add(x="Low State Timer (5 min)", y=w400) -> (x+y=w399:dbl)
        "Time Sum 1" <- w399
        n153 = Greater?(x=w406, y=w399) -> (0:w407:bool)
        n154 = case shown="True" w398 {
          tunnel: w411 -> [w421 w440]
          tunnel: [w420 w440] -> w410
          tunnel: [w419 "Wait for 35 Mins\nWait for 10 Mins\nData Process"] -> w409
          tunnel: w408 -> [w418 _]
          tunnel: w407 -> [w417 _]
          tunnel: w404 -> [w416 _]
          tunnel: string[] ["Time", "Power", "Ambient Temp (F)", "RH", "RDB (F)"] ("Array") -> [w415 _]
          frame False {
            n155 = case shown="False" w417 {
              tunnel: w421 -> [w430 w439]
              tunnel: [w429 w439] -> w420
              tunnel: [w427 "Wait 5 Min\nStabilize 5 Min\nOff Mode Collect 5 Min\nData Process" ("State(s) in Front (\"\")")] -> w419
              tunnel: w418 -> [w424 _]
              tunnel: w416 -> [w423 _]
              tunnel: w415 -> [w422 _]
              frame False {
                n156 = call "E-Time.vi"() -> ("Elapsed Time (sec)"=w431:dbl)  [unwired: 9 in, 2 out]
                n157 = call "RLT Timeout Calc.vi"("Complete time"=w431, "Gather Data Period"=1000, "Start Time"=w424) -> ("coerced(x)"=w426:i32)  [unwired: 8 in]
                n158 = event shown="[0] Timeout" {
                  selector: _ -> [_]
                  dyn-events: _ -> [_]
                  timeout: w426 -> [_]
                  tunnel: [w434] -> w428
                  tunnel: [w433] -> w427
                  tunnel: w423 -> [w432]
                  event Timeout {
                    n159 = event-data() -> ()  [unwired: 1 in, 2 out]
                    n160 = case shown="True" w432 {
                      tunnel: ["Post Time\nGet Power\nCheck for Low Power" ("State(s) in Front (\"\")") "" ("State(s) in Front (\"\")")] -> w433
                      frame True {
                      }
                      frame False {
                      }
                    }
                    n161 = call "E-Time.vi"() -> ("Elapsed Time (sec)"=w434:dbl)  [unwired: 9 in, 2 out]
                  }
                }
                n162 = Bundle By Name(cluster=w430, "Tstart"=w428, "Labels"=w422) -> (w429:T5)
              }
              frame True {
                n163 = local write "Low Power Switch"(FALSE ("Low Power Switch")) -> ()
              }
            }
          }
          frame True {
          }
        }
        n164 = local write "String"("Checking for a Low Power State...") -> ()
        n165 = call <vilib>:"Add State(s) to Queue__jki_lib_state_machine.vi"("State(s) in Front (\"\")"=w409, "State(s) in (\"\")"=w414) -> ("States Out"=w413:string)  [unwired: 13 in]
      }
      frame "Wait 5 Min" {
        # "Your code here.\n(You can make a copy of, or modify, this frame)"
        n166 = Unbundle By Name(w458) -> ("Tstart"=w455:dbl, "2015?"=w451:bool, "35 Min Data Array"=w449:dbl[])
        n167 = local read "Time Sum 1"() -> (w445:dbl)
        n168 = local read "Timer"() -> (w453:dbl)
        n169 = Add(x=w445, y="5 Min Timer") -> (x+y=w448:dbl)
        "Time Sum 3" <- w448
        n170 = Greater?(x=w453, y=w448) -> (0:w454:bool)
        n171 = Build Array (concatenate)(w443, w449) -> (w446:dbl[][])
        n172 = case shown="True" w454 {
          tunnel: w458 -> [w470 w481]
          tunnel: [w469 w481] -> w457
          tunnel: [w467 w477] -> w456
          tunnel: w455 -> [w464 _]
          tunnel: w451 -> [w463 _]
          tunnel: string[] ["Time", "Power", "Ambient Temp (F)", "RH", "RDB (F)"] ("Array") -> [w462 _]
          frame False {
            n173 = call "E-Time.vi"() -> ("Elapsed Time (sec)"=w471:dbl)  [unwired: 9 in, 2 out]
            n174 = call "RLT Timeout Calc.vi"("Complete time"=w471, "Gather Data Period"=1000, "Start Time"=w464) -> ("coerced(x)"=w466:i32)  [unwired: 8 in]
            n175 = event shown="[0] Timeout" {
              selector: _ -> [_]
              dyn-events: _ -> [_]
              timeout: w466 -> [_]
              tunnel: [w474] -> w468
              tunnel: [w473] -> w467
              tunnel: w463 -> [w472]
              event Timeout {
                n176 = event-data() -> ()  [unwired: 1 in, 2 out]
                n177 = case shown="True" w472 {
                  tunnel: ["Post Time\nGet Power\nWait 5 Min" ("State(s) in Front (\"\")") "" ("State(s) in Front (\"\")")] -> w473
                  frame True {
                  }
                  frame False {
                  }
                }
                n178 = call "E-Time.vi"() -> ("Elapsed Time (sec)"=w474:dbl)  [unwired: 9 in, 2 out]
              }
            }
            n179 = Bundle By Name(cluster=w470, "Tstart"=w468, "Labels"=w462) -> (w469:T5)
          }
          frame True {
            n180 = One Button Dialog(message="Turn Dryer Off", button name ("OK")="OK") -> (true=w478:bool)
            n181 = case shown="True" w478 {
              tunnel: ["Macro: Exit" ("State(s) in Front (\"\")") "" ("State(s) in Front (\"\")")] -> w477
              frame False {
              }
              frame True {
              }
            }
          }
        }
        n182 = local write "DOE Data"(w446) -> ()
        n183 = call <vilib>:"Add State(s) to Queue__jki_lib_state_machine.vi"("State(s) in Front (\"\")"=w456, "State(s) in (\"\")"=w461) -> ("States Out"=w460:string)  [unwired: 13 in]
        n184 = local write "String"("Collecting Standby Data For 5 Min...") -> ()
      }
      frame "Stabilize 5 Min" {
        # "Your code here.\n(You can make a copy of, or modify, this frame)"
        n185 = local read "Time Sum 3"() -> (w487:dbl)
        n186 = local read "5 Min Timer"() -> (w485:dbl)
        n187 = Unbundle By Name(w498) -> ("Tstart"=w495:dbl, "2015?"=w491:bool)
        n188 = local read "Timer"() -> (w493:dbl)
        n189 = Add(x=w487, y=w485) -> (x+y=w489:dbl)
        "Time Sum 4" <- w489
        n190 = Greater?(x=w493, y=w489) -> (0:w494:bool)
        n191 = case shown="True" w494 {
          tunnel: w498 -> [w510 w518]
          tunnel: [w509 w518] -> w497
          tunnel: [w507 "" ("State(s) in Front (\"\")")] -> w496
          tunnel: w495 -> [w504 _]
          tunnel: w491 -> [w503 _]
          tunnel: string[] ["Time", "Power", "Ambient Temp (F)", "RH", "RDB (F)"] ("Array") -> [w502 _]
          frame False {
            n192 = call "E-Time.vi"() -> ("Elapsed Time (sec)"=w511:dbl)  [unwired: 9 in, 2 out]
            n193 = call "RLT Timeout Calc.vi"("Complete time"=w511, "Gather Data Period"=1000, "Start Time"=w504) -> ("coerced(x)"=w506:i32)  [unwired: 8 in]
            n194 = event shown="[0] Timeout" {
              selector: _ -> [_]
              dyn-events: _ -> [_]
              timeout: w506 -> [_]
              tunnel: [w514] -> w508
              tunnel: [w513] -> w507
              tunnel: w503 -> [w512]
              event Timeout {
                n195 = event-data() -> ()  [unwired: 1 in, 2 out]
                n196 = case shown="True" w512 {
                  tunnel: ["Post Time\nGet Power\nStabilize 5 Min" ("State(s) in Front (\"\")") "" ("State(s) in Front (\"\")")] -> w513
                  frame True {
                  }
                  frame False {
                  }
                }
                n197 = call "E-Time.vi"() -> ("Elapsed Time (sec)"=w514:dbl)  [unwired: 9 in, 2 out]
              }
            }
            n198 = Bundle By Name(cluster=w510, "Tstart"=w508, "Labels"=w502) -> (w509:T5)
          }
          frame True {
          }
        }
        n199 = call <vilib>:"Add State(s) to Queue__jki_lib_state_machine.vi"("State(s) in Front (\"\")"=w496, "State(s) in (\"\")"=w501) -> ("States Out"=w500:string)  [unwired: 13 in]
        n200 = local write "String"("Stabilizing for 5 Min...") -> ()
      }
      frame "Off Mode Collect 5 Min" {
        # "Your code here.\n(You can make a copy of, or modify, this frame)"
        n201 = Unbundle By Name(w535) -> ("Tstart"=w532:dbl, "2015?"=w528:bool, "35 Min Data Array"=w525:dbl[])
        n202 = Build Array (concatenate)(w526, w525) -> (w521:dbl[][])
        n203 = local read "5 Min Timer"() -> (w520:dbl)
        n204 = local read "Time Sum 4"() -> (w523:dbl)
        n205 = local write "35 Min Data"(w521) -> ()
        n206 = local read "Timer"() -> (w530:dbl)
        n207 = Add(x=w520, y=w523) -> (x+y=w522:dbl)
        n208 = Greater?(x=w530, y=w522) -> (0:w531:bool)
        n209 = case shown="False" w531 {
          tunnel: w535 -> [w547 w555]
          tunnel: [w546 w555] -> w534
          tunnel: [w544 "" ("State(s) in Front (\"\")")] -> w533
          tunnel: w532 -> [w541 _]
          tunnel: w528 -> [w540 _]
          tunnel: string[] ["Time", "Power", "Ambient Temp (F)", "RH", "RDB (F)"] ("Array") -> [w539 _]
          frame False {
            n210 = call "E-Time.vi"() -> ("Elapsed Time (sec)"=w548:dbl)  [unwired: 9 in, 2 out]
            n211 = call "RLT Timeout Calc.vi"("Complete time"=w548, "Gather Data Period"=1000, "Start Time"=w541) -> ("coerced(x)"=w543:i32)  [unwired: 8 in]
            n212 = event shown="[0] Timeout" {
              selector: _ -> [_]
              dyn-events: _ -> [_]
              timeout: w543 -> [_]
              tunnel: [w551] -> w545
              tunnel: [w550] -> w544
              tunnel: w540 -> [w549]
              event Timeout {
                n213 = event-data() -> ()  [unwired: 1 in, 2 out]
                n214 = case shown="True" w549 {
                  tunnel: ["Post Time\nGet Power\nOff Mode Collect 5 Min" ("State(s) in Front (\"\")") "Post Time\nGet Power\nAgilent: Get Data\nWait for 5 Mins" ("State(s) in Front (\"\")")] -> w550
                  frame True {
                  }
                  frame False {
                  }
                }
                n215 = call "E-Time.vi"() -> ("Elapsed Time (sec)"=w551:dbl)  [unwired: 9 in, 2 out]
              }
            }
            n216 = Bundle By Name(cluster=w547, "Tstart"=w545, "Labels"=w539) -> (w546:T5)
          }
          frame True {
          }
        }
        n217 = local write "String"("Collecting Off Mode Watts...") -> ()
        n218 = call <vilib>:"Add State(s) to Queue__jki_lib_state_machine.vi"("State(s) in Front (\"\")"=w533, "State(s) in (\"\")"=w538) -> ("States Out"=w537:string)  [unwired: 13 in]
      }
      frame "Wait for 35 Mins" {
        # "Your code here.\n(You can make a copy of, or modify, this frame)"
        n219 = Unbundle By Name(w572) -> ("Tstart"=w569:dbl, "2015?"=w565:bool, "35 Min Data Array"=w562:dbl[])
        n220 = Build Array (concatenate)(w563, w562) -> (w561:dbl[][])
        "35 Min Data" <- w561
        n221 = local read "Time Sum 1"() -> (w558:dbl)
        n222 = local read "Timer"() -> (w567:dbl)
        n223 = Add(x="35 Min", y=w558) -> (x+y=w557:dbl)
        "Time Sum 2" <- w557
        n224 = Greater?(x=w567, y=w557) -> (0:w568:bool)
        n225 = case shown="False" w568 {
          tunnel: w572 -> [w584 w592]
          tunnel: [w583 w592] -> w571
          tunnel: [w581 "" ("State(s) in Front (\"\")")] -> w570
          tunnel: w569 -> [w578 _]
          tunnel: w565 -> [w577 _]
          tunnel: string[] ["Time", "Power", "Ambient Temp (F)", "RH", "RDB (F)"] ("Array") -> [w576 _]
          frame False {
            n226 = call "E-Time.vi"() -> ("Elapsed Time (sec)"=w585:dbl)  [unwired: 9 in, 2 out]
            n227 = call "RLT Timeout Calc.vi"("Complete time"=w585, "Gather Data Period"=1000, "Start Time"=w578) -> ("coerced(x)"=w580:i32)  [unwired: 8 in]
            n228 = event shown="[0] Timeout" {
              selector: _ -> [_]
              dyn-events: _ -> [_]
              timeout: w580 -> [_]
              tunnel: [w588] -> w582
              tunnel: [w587] -> w581
              tunnel: w577 -> [w586]
              event Timeout {
                n229 = event-data() -> ()  [unwired: 1 in, 2 out]
                n230 = case shown="True" w586 {
                  tunnel: ["Post Time\nGet Power\nWait for 35 Mins" ("State(s) in Front (\"\")") "Post Time\nGet Power\nAgilent: Get Data\nWait for 5 Mins" ("State(s) in Front (\"\")")] -> w587
                  frame True {
                  }
                  frame False {
                  }
                }
                n231 = call "E-Time.vi"() -> ("Elapsed Time (sec)"=w588:dbl)  [unwired: 9 in, 2 out]
              }
            }
            n232 = Bundle By Name(cluster=w584, "Tstart"=w582, "Labels"=w576) -> (w583:T5)
          }
          frame True {
          }
        }
        n233 = local write "String"("Off Mode Stabilization...") -> ()
        n234 = call <vilib>:"Add State(s) to Queue__jki_lib_state_machine.vi"("State(s) in Front (\"\")"=w570, "State(s) in (\"\")"=w575) -> ("States Out"=w574:string)  [unwired: 13 in]
      }
      frame "Wait for 10 Mins" {
        # "Your code here.\n(You can make a copy of, or modify, this frame)"
        n235 = Unbundle By Name(w609) -> ("Tstart"=w606:dbl, "2015?"=w602:bool, "35 Min Data Array"=w600:dbl[])
        n236 = local read "Time Sum 2"() -> (w595:dbl)
        n237 = Build Array (concatenate)(w599, w600) -> (w598:dbl[][])
        "DOE Data" <- w598
        n238 = local read "Timer"() -> (w604:dbl)
        n239 = Add(x="10 Min Power", y=w595) -> (x+y=w596:dbl)
        n240 = Greater?(x=w604, y=w596) -> (0:w605:bool)
        n241 = case shown="False" w605 {
          tunnel: w609 -> [w621 w629]
          tunnel: [w620 w629] -> w608
          tunnel: [w618 "" ("State(s) in Front (\"\")")] -> w607
          tunnel: w606 -> [w615 _]
          tunnel: w602 -> [w614 _]
          tunnel: string[] ["Time", "Power", "Ambient Temp (F)", "RH", "RDB (F)"] ("Array") -> [w613 _]
          frame False {
            n242 = call "E-Time.vi"() -> ("Elapsed Time (sec)"=w622:dbl)  [unwired: 9 in, 2 out]
            n243 = call "RLT Timeout Calc.vi"("Complete time"=w622, "Gather Data Period"=1000, "Start Time"=w615) -> ("coerced(x)"=w617:i32)  [unwired: 8 in]
            n244 = event shown="[0] Timeout" {
              selector: _ -> [_]
              dyn-events: _ -> [_]
              timeout: w617 -> [_]
              tunnel: [w625] -> w619
              tunnel: [w624] -> w618
              tunnel: w614 -> [w623]
              event Timeout {
                n245 = event-data() -> ()  [unwired: 1 in, 2 out]
                n246 = case shown="True" w623 {
                  tunnel: ["Post Time\nGet Power\nWait for 10 Mins" ("State(s) in Front (\"\")") "Post Time\nGet Power\nAgilent: Get Data\nWait for 5 Mins" ("State(s) in Front (\"\")")] -> w624
                  frame True {
                  }
                  frame False {
                  }
                }
                n247 = call "E-Time.vi"() -> ("Elapsed Time (sec)"=w625:dbl)  [unwired: 9 in, 2 out]
              }
            }
            n248 = Bundle By Name(cluster=w621, "Tstart"=w619, "Labels"=w613) -> (w620:T5)
          }
          frame True {
          }
        }
        n249 = local write "String"("Collecting Data For 10 Min...") -> ()
        n250 = call <vilib>:"Add State(s) to Queue__jki_lib_state_machine.vi"("State(s) in Front (\"\")"=w607, "State(s) in (\"\")"=w612) -> ("States Out"=w611:string)  [unwired: 13 in]
      }
      frame "Data Process" {
        # "Your code here.\n(You can make a copy of, or modify, this frame)"
        n251 = Unbundle By Name(w631) -> ("Output Data"=w650:T6)
        n252 = local read "Low Power Switch"() -> (w637:bool)
        n253 = case shown="False" w637 {
          tunnel: [w668 w686] -> w655
          tunnel: [w670 w691] -> w654
          tunnel: [w665 w686] -> w653
          tunnel: [w667 w686] -> w652
          tunnel: [w666 w686] -> w651
          tunnel: [w673 w690] -> w635
          tunnel: [w669 w689] -> w649
          tunnel: [w671 w688] -> w648
          tunnel: [w672 w687] -> w647
          frame False {
            # "Due to the order of the state machine, \nI had to switch the order of the  standby\nand off mode values."
            n254 = local read "DOE Data"() -> (w680:dbl[][])
            n255 = local read "35 Min Data"() -> (w681:dbl[][])
            n256 = Delete From Array(array=w680, index (col)=1 ("disabled index (col)")) -> (deleted portion=w677:dbl[])  [unwired: 2 in, 1 out]
            n257 = Delete From Array(array=w681, index (col)=1 ("disabled index (col)")) -> (deleted portion=w685:dbl[])  [unwired: 2 in, 1 out]
            n258 = call <vilib>:"Histogram.vi"("X"=w677) -> ("Histogram Graph"=w676:T1)  [unwired: 7 in, 3 out]
            n259 = call <vilib>:"Std Deviation and Variance.vi"("X"=w677) -> ("mean"=w668:dbl, "standard deviation"=w665:dbl)  [unwired: 1 in, 1 out]
            n260 = Array Max & Min(array=w677) -> (max value=w667:dbl)  [unwired: 3 out]
            n261 = call <vilib>:"Histogram.vi"("X"=w685) -> ("Histogram Graph"=→"Standby Mode Watts":T1)  [unwired: 7 in, 3 out]
            n262 = call <vilib>:"Std Deviation and Variance.vi"("X"=w685) -> ("mean"=w670:dbl, "standard deviation"=w669:dbl)  [unwired: 1 in, 1 out]
            n263 = Array Max & Min(array=w685) -> (max value=w671:dbl)  [unwired: 3 out]
            n264 = local write "Off Mode Watts"(w676) -> ()
            n265 = Multiply(x=w667, y=0.05) -> (x*y=w666:dbl)
            n266 = Multiply(x=w671, y=0.05) -> (x*y=w672:dbl)
            n267 = Less?(x=w665, y=w666) -> (x < y?=w675:bool)
            n268 = Less?(x=w669, y=w672) -> (x < y?=w674:bool)
            n269 = And(x=w675, y=w674) -> (x .and. y?=w673:bool)
          }
          frame True {
            w686 = 0.0
            n270 = local read "DOE Data"() -> (w696:dbl[][])
            n271 = Delete From Array(array=w696, index (col)=1 ("disabled index (col)")) -> (deleted portion=w692:dbl[])  [unwired: 2 in, 1 out]
            n272 = call <vilib>:"Std Deviation and Variance.vi"("X"=w692) -> ("mean"=w691:dbl, "standard deviation"=w689:dbl)  [unwired: 1 in, 1 out]
            n273 = Array Max & Min(array=w692) -> (max value=w688:dbl)  [unwired: 3 out]
            n274 = call <vilib>:"Histogram.vi"("X"=w692) -> ("Histogram Graph"=→"Off Mode Watts":T1)  [unwired: 7 in, 3 out]
            n275 = Multiply(x=w688, y=0.05) -> (x*y=w687:dbl)
            n276 = Less?(x=w689, y=w687) -> (x < y?=w690:bool)
          }
        }
        "Stable?" <- w635
        n277 = Bundle By Name(cluster=w650, "Standard Deviation"=w653, "Off Mode Watts"=w654, "Standby Watts"=w655, "Max Value"=w652, "5% of Max"=w651, "Standard Deviation."=w649, "Max Value."=w648, "5% of Max."=w647) -> (w646:T6)
        n278 = Unbundle By Name(w646) -> ("Off Mode Watts"=→"Off Mode Watts":dbl, "Standard Deviation."=→"Standard Deviation.":dbl, "Max Value."=→"Max Value.":dbl, "5% of Max."=→"5% of Max.":dbl, "Standby Watts"=→"Standby Watts":dbl, "Standard Deviation"=→"Standard Deviation":dbl, "Max Value"=→"Max Value":dbl, "5% of Max"=→"5% of Max":dbl)
        n279 = local write "Main Tab"(enum32{"Collecting", "Analyzed"}."Analyzed" ("Main Tab")) -> ()
        n280 = local write "Processed Data"(TRUE ("Processed Data")) -> ()
        n281 = Equal?(x=w635, y=FALSE) -> (x = y?=w633:bool)
        n282 = case shown="False" w633 {
          frame False {
            w663 = TRUE ("Visible")
            n283 = property on="Complete Test" class="Bool (strict)"("Visible"=w663) -> ()  [unwired: 2 in, 2 out]
            "Complete?" <- w663
          }
          frame True {
            w664 = TRUE ("Visible")
            n284 = property on="Complete Test" class="Bool (strict)"("Visible"=w664) -> ()  [unwired: 2 in, 2 out]
            n285 = property on="Restart" class="Bool (strict)"("Visible"=w664) -> ()  [unwired: 2 in, 2 out]
          }
        }
        n286 = local write "String"("Processing Data...") -> ()
        n287 = call <vilib>:"Add State(s) to Queue__jki_lib_state_machine.vi"("State(s) in Front (\"\")"="", "State(s) in (\"\")"=w662) -> ("States Out"=w661:string)  [unwired: 13 in]
      }
      frame "Init: Time" {
        # "Your code here.\n(You can make a copy of, or modify, this frame)"
        n288 = call "E-Time.vi"("error in (no error)"=w700) -> ("error out"=w702:errorcluster, "Elapsed Time (sec)"=w703:dbl)  [unwired: 8 in, 1 out]
        n289 = Bundle By Name(cluster=w701, "T0"=w703, "Tstart"=w703) -> (w704:T5)
        n290 = call <vilib>:"Add State(s) to Queue__jki_lib_state_machine.vi"("State(s) in (\"\")"=w706) -> ("States Out"=w705:string)  [unwired: 14 in]
      }
      frame "Get Power" {
        # "If the power drops below\n75% of the High Power.\nConsider that the low\npower state"
        # "Your code here.\n(You can make a copy of, or modify, this frame)"
        n291 = Unbundle By Name(w724) -> ("2015?"=w719:bool, "35 Min Data Array"=w722:dbl[], "Remote Port"=w707:i32, "Aplus IP Address"=w708:string)
        n292 = case shown="False" "Testing" {
          tunnel: [w732 "Test Power"] -> w714
          tunnel: w719 -> [_ _]
          tunnel: w718 -> [w730 w733]
          tunnel: [w729 w733] -> w717
          tunnel: w708 -> [w728 _]
          tunnel: w707 -> [w727 _]
          frame False {
            n293 = call "APLUS Camille Bauer Driver.vi"("error in (no error)"=w730, "Remote Port"=w727, "Remote IP Address"=w728) -> ("error out"=w729:errorcluster, "output cluster"=w731:T8)  [unwired: 7 in]
            n294 = Unbundle By Name(w731) -> ("Power"=w732:sgl)
          }
          frame True {
          }
        }
        "Power (Watts)" <- w714
        "Power Chart" <- w714
        n295 = Build Array (concatenate)(w722, w714) -> (w721:dbl[])
        n296 = local read "High Power"() -> (w710:dbl)
        n297 = call <vilib>:"Add State(s) to Queue__jki_lib_state_machine.vi"("State(s) in (\"\")"=w726) -> ("States Out"=w725:string)  [unwired: 14 in]
        n298 = Multiply(x=w710, y=0.75) -> (x*y=w709:dbl)
        n299 = Less?(x=w714, y=w709) -> (x < y?=w713:bool)
        n300 = Bundle By Name(cluster=w724, "35 Min Data Array"=w721, "Low Power State?"=w713) -> (w723:T5)
      }
      frame "Post Time" {
        # "Your code here.\n(You can make a copy of, or modify, this frame)"
        n301 = Unbundle By Name(w741) -> ("T0"=w743:dbl)
        n302 = call "E-Time.vi"() -> ("Elapsed Time (sec)"=w744:dbl)  [unwired: 9 in, 2 out]
        n303 = Subtract(x=w744, y=w743) -> (x-y=w739:dbl)
        "Timer" <- w739
        n304 = Build Array(w739) -> (w738:dbl[])
        n305 = Bundle By Name(cluster=w741, "35 Min Data Array"=w738) -> (w740:T5)
        n306 = call <vilib>:"Add State(s) to Queue__jki_lib_state_machine.vi"("State(s) in (\"\")"=w746) -> ("States Out"=w745:string)  [unwired: 14 in]
      }
    }
    n307 = case shown="True" "Debug?" {
      tunnel: w37 -> [_ w57]
      tunnel: w35 -> [w54 w56]
      tunnel: [w54 w55] -> w36
      frame False {
      }
      frame True {
        n308 = Build Array (concatenate)(w56, w57) -> (w55:string[])
        "Debug State" <- w55
      }
    }
    n309 = case shown="True" "stop" {
      tunnel: [w48 w53] -> w29
      tunnel: w30 -> [w48 w50]
      frame False {
      }
      frame True {
        n310 = call <vilib>:"Add State(s) to Queue__jki_lib_state_machine.vi"("State(s) in Front (\"\")"="Macro: Exit", "State(s) in (\"\")"=w50) -> ("States Out"=w53:string)  [unwired: 13 in]
        n311 = local write "Skip Standby"(FALSE ("Exit")) -> ()
        n312 = local write "Complete?"(TRUE ("Complete?")) -> ()
      }
    }
  }
  "Error Out" <- w5
